vi "Update_Analized_Overlay.vi"(4 "Color":u32(colorbox)=16711680, 6 "Index":i32, 7 "ROI Entry":T11={"vROIName"="", "vROIContour"={"Contour Type"=0, "ROI Type"=0, "Points"=[]}, "ProcessSetting"=[], "Analysis_Setting"={"PreProcess"=enum."*Algorithm*", "Parameter"=""}}, 8 "error in (no error)":errorcluster, 9 "DLL/Vision":bool, 10 "AnalysisResult":variant, 11 "Image Refnum":refnum<vi>) -> (0 "error out":errorcluster, 3 "DLL Vision_Image":T7)   [LabVIEW 2019]
uses:
  DLL/[Global] Image.vi
  <vilib>/vision/NI_Vision_Development_Module.lvlib
  Analysis/Controls/Parttern Match/Analysis_PatternMatch_ResultWithnumber.ctl
  Analysis/Controls/Contour/Analysis_Contour_Result.ctl
  Analysis/Controls/ColorMatch/Analysis_ColorMatch_Result.ctl
  Process/Controls/Process_Setting.ctl
  Analysis/Controls/Analysis_Setting.ctl
  Controls/Vision_DataEntry.ctl
  <vilib>/vision/Measure.llb/Edge New.ctl
  <vilib>/vision/Image Controls.llb/IMAQ Image.ctl
  Ctrl/VisionProcessName.ctl
panel:
  in  "data":T1
  in  "Particle Cluster":T2
  in  "output cluster":T3
  in  "Clamp Cluster":T4={"Points"=[], "Perpendicular Lines"=[], "appended array"=[], "Line Coordinates"=[], "Clamp Settings"={"Contrast"=0, "Filter width"=0, "Steepness"=0, "Subsampling Ratio"=0, "Show Search Area"=FALSE, "Show Search Lines"=FALSE, "Show Edges Found"=FALSE, "Show Result"=FALSE}, "ROI Descriptor"={"Global Rectangle"=[], "Contours"=[]}, "Distance"=0.0, "Edge Coordinates"=[{"X"=441.67966, "Y"=663.0}, {"X"=684.4586, "Y"=655.0}], "Edge Coordinates  (Real World)"=[{"X"=441.67966, "Y"=663.0}, {"X"=684.4586, "Y"=655.0}], "Distance (Real World)"=0.0}
  in  "Edge Detectionoutput cluster":T6 {"Edge Information"."Distance (Real-World)" format="%.2f"; "Edge Information"."Location (Real-World)"."Y" format="%.2g"; "Edge Information"."Location (Real-World)"."X" format="%.2f"; "Edge Information"."Noise" format="%.2f"; "Edge Information"."Location (Pixel)"."Y" format="%.2g"; "Edge Information"."Location (Pixel)"."X" format="%.2f"; "Edge Information"."Strength" format="%.2f"; "Edge Information"."Distance (Pixel)" format="%.2f"}
  in  "Straight Edge Cluster Array":T8(array[cluster])
  in  "Barcode 1D output cluster":T9
  in  "Barcode 2D output cluster":T10
  in  "Vision_Image":T7(plugin-control)
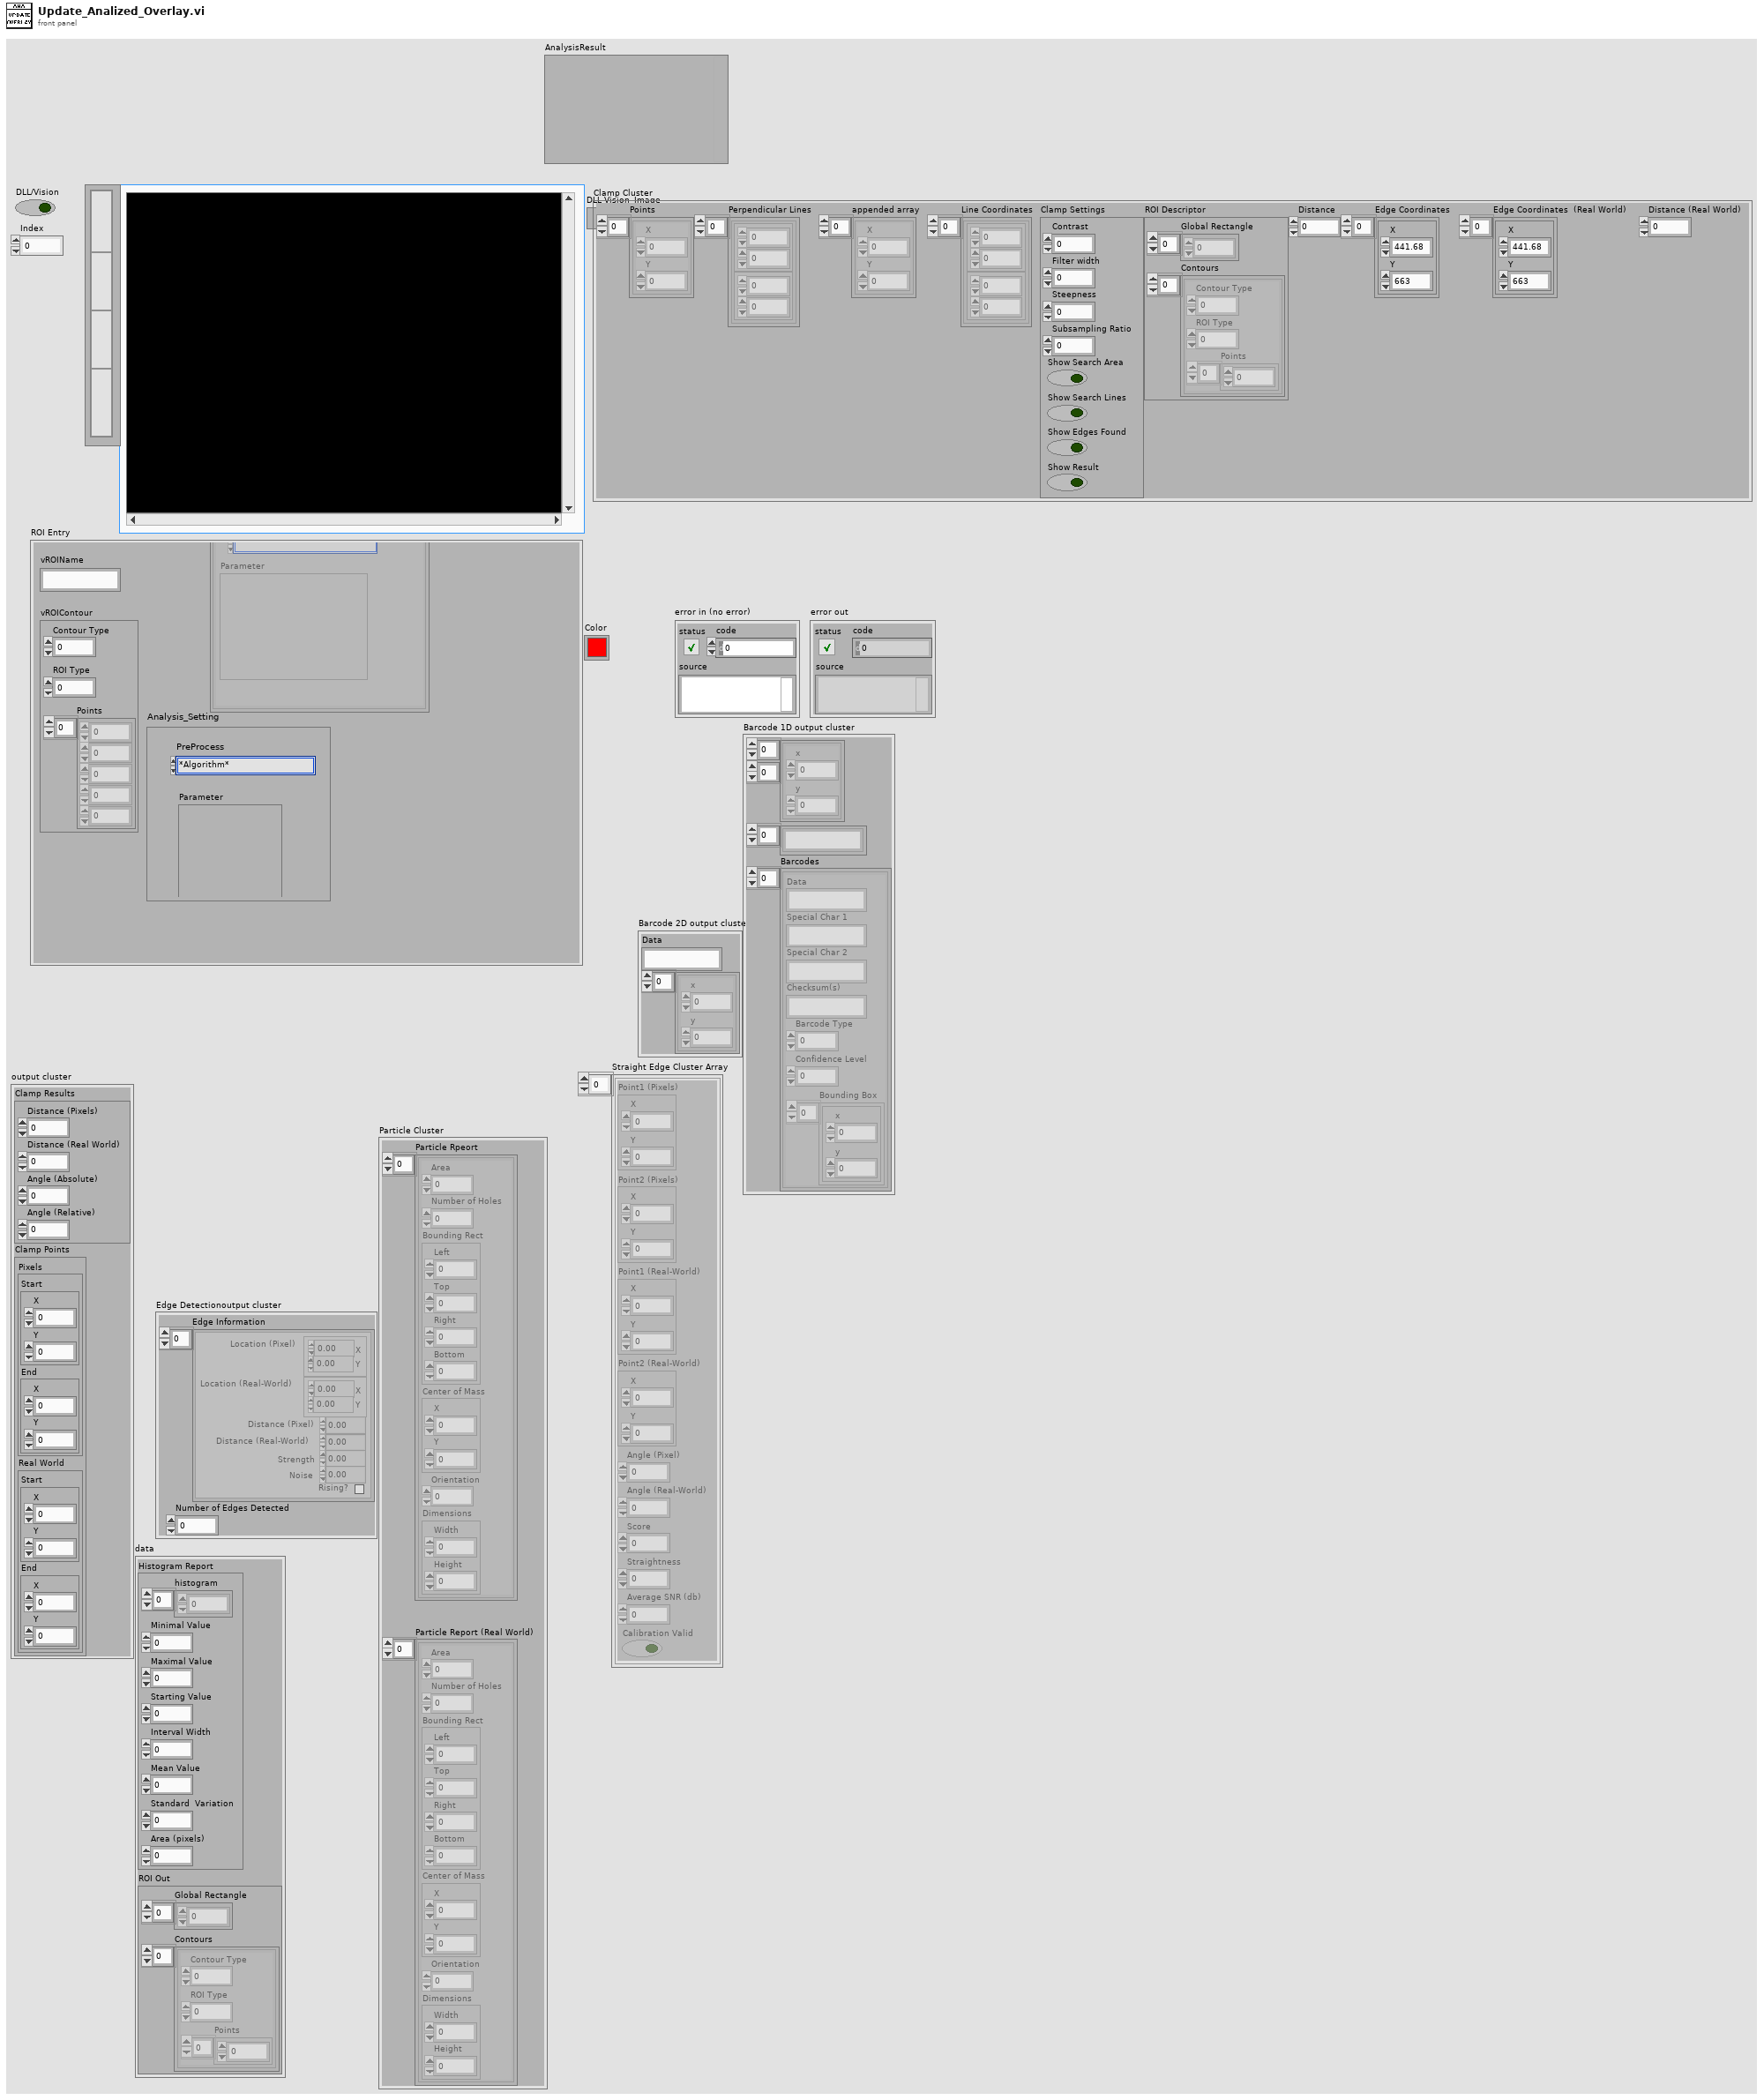
[diagram p1: front panel]
types:
  T1 = cluster{"Histogram Report":cluster{"histogram":u32[], "Minimal Value":sgl, "Maximal Value":sgl, "Starting Value":sgl, "Interval Width":sgl, "Mean Value":sgl, "Standard  Variation":sgl, "Area (pixels)":i32}, "ROI Out":cluster{"Global Rectangle":i32[], "Contours":cluster{"Contour Type":u32, "ROI Type":u32, "Points":i32[]}[]}}
  T2 = cluster{"Particle Rpeort":cluster{"Area":dbl, "Number of Holes":dbl, "Bounding Rect":cluster{"Left":dbl, "Top":dbl, "Right":dbl, "Bottom":dbl}, "Center of Mass":cluster{"X":dbl, "Y":dbl}, "Orientation":dbl, "Dimensions":cluster{"Width":dbl, "Height":dbl}}[], "Particle Report (Real World)":cluster{"Area":dbl, "Number of Holes":dbl, "Bounding Rect":cluster{"Left":dbl, "Top":dbl, "Right":dbl, "Bottom":dbl}, "Center of Mass":cluster{"X":dbl, "Y":dbl}, "Orientation":dbl, "Dimensions":cluster{"Width":dbl, "Height":dbl}}[]}
  T3 = cluster{"Clamp Results":cluster{"Distance (Pixels)":dbl, "Distance (Real World)":dbl, "Angle (Absolute)":dbl, "Angle (Relative)":dbl}, "Clamp Points":cluster{"Pixels ":cluster{"Start":cluster{"X":dbl, "Y":dbl}, "End":cluster{"X":dbl, "Y":dbl}}, "Real World":cluster{"Start":cluster{"X":dbl, "Y":dbl}, "End":cluster{"X":dbl, "Y":dbl}}}}
  T4 = cluster{"Points":cluster{"X":sgl, "Y":sgl}[], "Perpendicular Lines":cluster{cluster{sgl, sgl}, cluster{sgl, sgl}}[], "appended array":cluster{"X":sgl, "Y":sgl}[], "Line Coordinates":cluster{cluster{sgl, sgl}, cluster{sgl, sgl}}[], "Clamp Settings":cluster{"Contrast":i32, "Filter width":i32, "Steepness":i32, "Subsampling Ratio":u32, "Show Search Area":bool, "Show Search Lines":bool, "Show Edges Found":bool, "Show Result":bool}, "ROI Descriptor":cluster{"Global Rectangle":i32[], "Contours":cluster{"Contour Type":u32, "ROI Type":u32, "Points":i32[]}[]}, "Distance":sgl, "Edge Coordinates":cluster{"X":sgl, "Y":sgl}[], "Edge Coordinates  (Real World)":cluster{"X":sgl, "Y":sgl}[], "Distance (Real World)":sgl}
  T5 = typedef "Edge New.ctl" = cluster{"Location (Pixel)":cluster{"X":sgl, "Y":sgl}, "Location (Real-World)":cluster{"X":sgl, "Y":sgl}, "Distance (Pixel)":dbl, "Distance (Real-World)":dbl, "Strength":dbl, "Noise":dbl, "Rising?":bool}
  T6 = cluster{"Edge Information":T5[], "Number of Edges Detected":i32}
  T7 = typedef "IMAQ Image.ctl" = refnum<image>
  T8 = cluster{"Point1 (Pixels)":cluster{"X":sgl, "Y":sgl}, "Point2 (Pixels)":cluster{"X":sgl, "Y":sgl}, "Point1 (Real-World)":cluster{"X":sgl, "Y":sgl}, "Point2 (Real-World)":cluster{"X":sgl, "Y":sgl}, "Angle (Pixel)":dbl, "Angle (Real-World)":dbl, "Score":dbl, "Straightness":dbl, "Average SNR (db)":dbl, "Calibration Valid":bool}[]
  T9 = cluster{cluster{"x":sgl, "y":sgl}[][], string[], "Barcodes":cluster{"Data":string, "Special Char 1":string, "Special Char 2":string, "Checksum(s)":string, "Barcode Type":u32, "Confidence Level":sgl, "Bounding Box":cluster{"x":sgl, "y":sgl}[]}[]}
  T10 = cluster{"Data":string, cluster{"x":sgl, "y":sgl}[]}
  T11 = typedef "Vision_DataEntry.ctl" = cluster{"vROIName":string, "vROIContour":cluster{"Contour Type":u32, "ROI Type":u32, "Points":i32[]}, "ProcessSetting":T12[], "Analysis_Setting":T14}
  T12 = typedef "Process_Setting.ctl" = cluster{"Enum_PreProcess":T13, "Parameter":string}
  T13 = typedef "VisionProcessName.ctl" = enum16{"*CamParameter*", "CamAttributes", "*Preprocess*", "CG_Brightness", "C_Plane Extraction", "C_Threshold", "G_Lookup Table", "G_Threshold"}
  T14 = typedef "Analysis_Setting.ctl" = cluster{"PreProcess":T15, "Parameter":string}
  T15 = typedef "VisionProcessName.ctl" = enum16{"*CamParameter*", "CamAttributes", "*Preprocess*", "CG_Brightness", "C_Plane Extraction", "C_Threshold", "G_Lookup Table", "G_Threshold", "B_Image Inversion", "*Algorithm*", "CG_Histogram", "C_Color Matching", "C_Color Pattern Matching", "G_PatternMatch", "CG_Find Straight Edge", "CG_Adv. Find Straight Edge", "CG_Find Circular Edge", "G_Max Clamp", "G_Clamp (Rake)", "G_Pattern Matching"}
  T16 = typedef "Analysis_Type.ctl" = u16
  T17 = typedef "Analysis_PatternMatch_ResultWithnumber.ctl" = cluster{"numbers":i32, "results":cluster{"ROI Descriptor out":T18, "Point":T19, "Angle":sgl, "Score":sgl, "Real World Coordinates":cluster{"X":sgl, "Y":sgl}, "Rectangle":T20}[]}
  T18 = typedef "ROI Descriptor" = cluster{"Global Rectangle":i32[], "Contours":cluster{"ID":enum32{"External", "Internal"}, "Type":u32, "Coordinates":i32[]}[]}
  T19 = typedef "IMAQ Point" = cluster{"X":sgl, "Y":sgl}
  T20 = typedef "IMAQ Rectangle" = cluster{"Left":i32, "Top":i32, "Right":i32, "Bottom":i32, "Rotation":dbl}
  T21 = cluster{"ROI Descriptor out":T18, "ROI Descriptor out":T18, "Fitted Circle":cluster{"Center (Pixels)":cluster{"X":sgl, "Y":sgl}, "Radius (Pixels)":dbl, "Center (Real-World)":cluster{"X":sgl, "Y":sgl}, "Radius (Real-World)":dbl, "Roundness (Real-World)":dbl, "Average Strength":dbl, "Average SNR (dB)":dbl}}
  T22 = cluster{"Desired Font (Application)":enum16{"User-specified Font", "Application Font", "System Font", "Dialog Font"}, "[User-specified Font]":cluster{"Font Name":string, "Size":i16, "Strikeout?":bool, "Italic?":bool, "Underline?":bool, "Outline?":bool, "Shadow?":bool, "Bold?":bool, "Rotation Angle":dbl}, "Horizontal Alignment":i16, "Vertical Alignment":i16}
  T23 = typedef "Analysis_Contour_Result.ctl" = cluster{"Points (pixel)":cluster{"X":dbl, "Y":dbl}[], "Points (real)":cluster{"X":dbl, "Y":dbl}[], "Length (pixel)":dbl, "Length (real)":dbl}
  T24 = typedef "Analysis_ColorMatch_Result.ctl" = cluster{"Match Flag":bool[], "Match Score":i32[], "ROI Descriptor":T18}
  T25 = cluster{"ROI Descriptor out":T18, "Point":T19, "Angle":sgl, "Score":sgl, "Real World Coordinates":cluster{"X":sgl, "Y":sgl}, "Rectangle":T20}[]
  T26 = cluster{"Contrast":i32, "Filter width":i32, "Steepness":i32, "Subsampling Ratio":u32, "Show Search Area":bool, "Show Search Lines":bool, "Show Edges Found":bool, "Show Result":bool}
  T27 = cluster{"Global Rectangle":i32[], "Contours":cluster{"Contour Type":u32, "ROI Type":u32, "Points":i32[]}[]}
  T28 = cluster{"Start":cluster{"X":dbl, "Y":dbl}, "End":cluster{"X":dbl, "Y":dbl}}
  T29 = cluster{"End":cluster{"X":dbl, "Y":dbl}, "Start":cluster{"X":dbl, "Y":dbl}}
  T30 = cluster{"Point 1":cluster{"X":sgl, "Y":sgl}, "Point 2":cluster{"X":sgl, "Y":sgl}}
  T31 = cluster{cluster{sgl, sgl}, "End":cluster{"X":dbl, "Y":dbl}}
  T32 = cluster{cluster{sgl, sgl}, "Start":cluster{"X":dbl, "Y":dbl}}
  T33 = cluster{"Point 1":cluster{"X":sgl, "Y":sgl}, "Point 2":cluster{"X":sgl, "Y":sgl}}[]
  T34 = cluster{cluster{"X":dbl, "Y":dbl}, cluster{"X":dbl, "Y":dbl}}
  T35 = cluster{cluster{"X":dbl, "Y":dbl}, "End":cluster{"X":dbl, "Y":dbl}}
  T36 = cluster{cluster{"X":dbl, "Y":dbl}, "Start":cluster{"X":dbl, "Y":dbl}}
  T37 = cluster{cluster{"X":dbl, "Y":dbl}, cluster{"X":dbl, "Y":dbl}}[]
  T38 = cluster{"Area":dbl, "Number of Holes":dbl, "Bounding Rect":cluster{"Left":dbl, "Top":dbl, "Right":dbl, "Bottom":dbl}, "Center of Mass":cluster{"X":dbl, "Y":dbl}, "Orientation":dbl, "Dimensions":cluster{"Width":dbl, "Height":dbl}}[]
  T39 = cluster{"Left":dbl, "Top":dbl, "Right":dbl, "Bottom":dbl}
  T40 = cluster{"Contour Type":u32, "ROI Type":u32, "Points":i32[]}[]
  T41 = cluster{"Contour Type":u32, "ROI Type":u32, "Points":i32[]}
  T42 = cluster{"Enum_ShapeType":enum16{"Circles", "Ellipses", "Lines", "Rectangles"}, "numbers":i32, "ReAnfle":cluster{"Rectangle Descriptor":cluster{"Corners":cluster{"X":sgl, "Y":sgl}[], "Angle":dbl, "Width":dbl, "Height":dbl, "Score":dbl}, "Rectangle Descriptor(Real)":cluster{"Corners":cluster{"X":sgl, "Y":sgl}[], "Angle":dbl, "Width":dbl, "Height":dbl, "Score":dbl}}[]}
  T43 = cluster{"Enum_ShapeType":enum16{"Circles", "Ellipses", "Lines", "Rectangles"}, "numbers":i32, "Lines":cluster{"Circle Descriptor":cluster{"Start Point":cluster{"X":sgl, "Y":sgl}, "End Point":cluster{"X":sgl, "Y":sgl}, "Length":dbl, "Angle":dbl, "Score":dbl}, "Circle Descriptor(Real)":cluster{"Start Point":cluster{"X":sgl, "Y":sgl}, "End Point":cluster{"X":sgl, "Y":sgl}, "Length":dbl, "Orientation":dbl, "Score":dbl}}[]}
  T44 = cluster{"Enum_ShapeType":enum16{"Circles", "Ellipses", "Lines", "Rectangles"}, "numbers":i32, "Ellipse":cluster{"ROI Descriptor out":T18, "Circle Descriptor":cluster{"Position":cluster{"X":sgl, "Y":sgl}, "Angle":dbl, "Major Radius":dbl, "Minor Radius":dbl, "Score":dbl}, "Circle Descriptor(Real)":cluster{"Position":cluster{"X":sgl, "Y":sgl}, "Orientation":dbl, "Major Radius":dbl, "Minor Radius":dbl, "Score":dbl}}[]}
  T45 = cluster{"Enum_ShapeType":enum16{"Circles", "Ellipses", "Lines", "Rectangles"}, "numbers":i32, "Circle ":cluster{"ROI Descriptor out":T18, "Circle Descriptor":cluster{"Position":cluster{"X":sgl, "Y":sgl}, "Radius":dbl, "Score":dbl}, "Circle Descriptor(Real)":cluster{"Position":cluster{"X":sgl, "Y":sgl}, "Radius":dbl, "Score":dbl}}[]}
  T46 = cluster{"ROI Descriptor out":T18, "Circle Descriptor":cluster{"Position":cluster{"X":sgl, "Y":sgl}, "Radius":dbl, "Score":dbl}, "Circle Descriptor(Real)":cluster{"Position":cluster{"X":sgl, "Y":sgl}, "Radius":dbl, "Score":dbl}}[]
  T47 = cluster{"ROI Descriptor out":T18, "Circle Descriptor":cluster{"Position":cluster{"X":sgl, "Y":sgl}, "Angle":dbl, "Major Radius":dbl, "Minor Radius":dbl, "Score":dbl}, "Circle Descriptor(Real)":cluster{"Position":cluster{"X":sgl, "Y":sgl}, "Orientation":dbl, "Major Radius":dbl, "Minor Radius":dbl, "Score":dbl}}[]
  T48 = cluster{"Position":cluster{"X":sgl, "Y":sgl}, "Angle":dbl, "Major Radius":dbl, "Minor Radius":dbl, "Score":dbl}
  T49 = cluster{dbl, dbl, "Major Radius":dbl, "Minor Radius":dbl}
  T50 = cluster{"Circle Descriptor":cluster{"Start Point":cluster{"X":sgl, "Y":sgl}, "End Point":cluster{"X":sgl, "Y":sgl}, "Length":dbl, "Angle":dbl, "Score":dbl}, "Circle Descriptor(Real)":cluster{"Start Point":cluster{"X":sgl, "Y":sgl}, "End Point":cluster{"X":sgl, "Y":sgl}, "Length":dbl, "Orientation":dbl, "Score":dbl}}[]
  T51 = cluster{"Start Point":cluster{"X":sgl, "Y":sgl}, "End Point":cluster{"X":sgl, "Y":sgl}, "Length":dbl, "Angle":dbl, "Score":dbl}
  T52 = cluster{"Rectangle Descriptor":cluster{"Corners":cluster{"X":sgl, "Y":sgl}[], "Angle":dbl, "Width":dbl, "Height":dbl, "Score":dbl}, "Rectangle Descriptor(Real)":cluster{"Corners":cluster{"X":sgl, "Y":sgl}[], "Angle":dbl, "Width":dbl, "Height":dbl, "Score":dbl}}[]
  T53 = cluster{"Corners":cluster{"X":sgl, "Y":sgl}[], "Angle":dbl, "Width":dbl, "Height":dbl, "Score":dbl}
  T54 = cluster{"ID":enum32{"External", "Internal"}, "Type":u32, "Coordinates":i32[]}[]
  T55 = cluster{"Coordinates[0]":i32, "Coordinates[1]":i32}
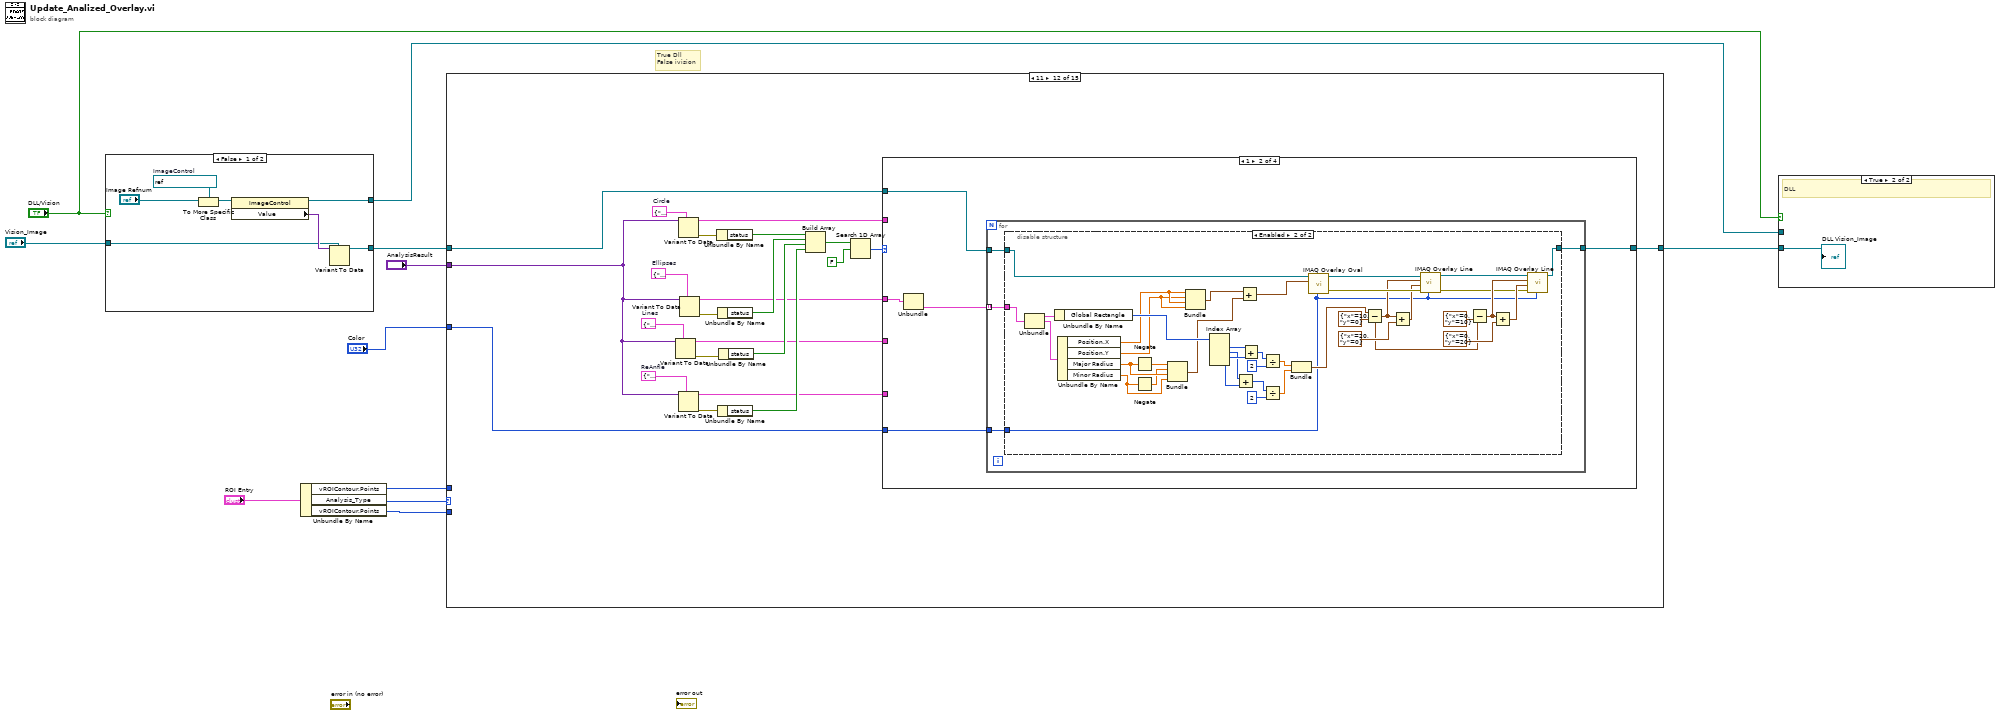
[diagram p0: block diagram]
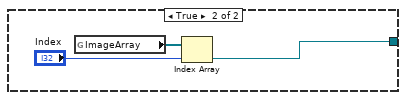
[diagram p2: hidden frame]
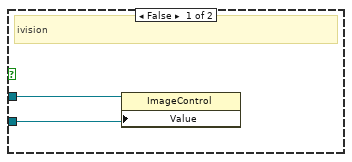
[diagram p3: hidden frame]
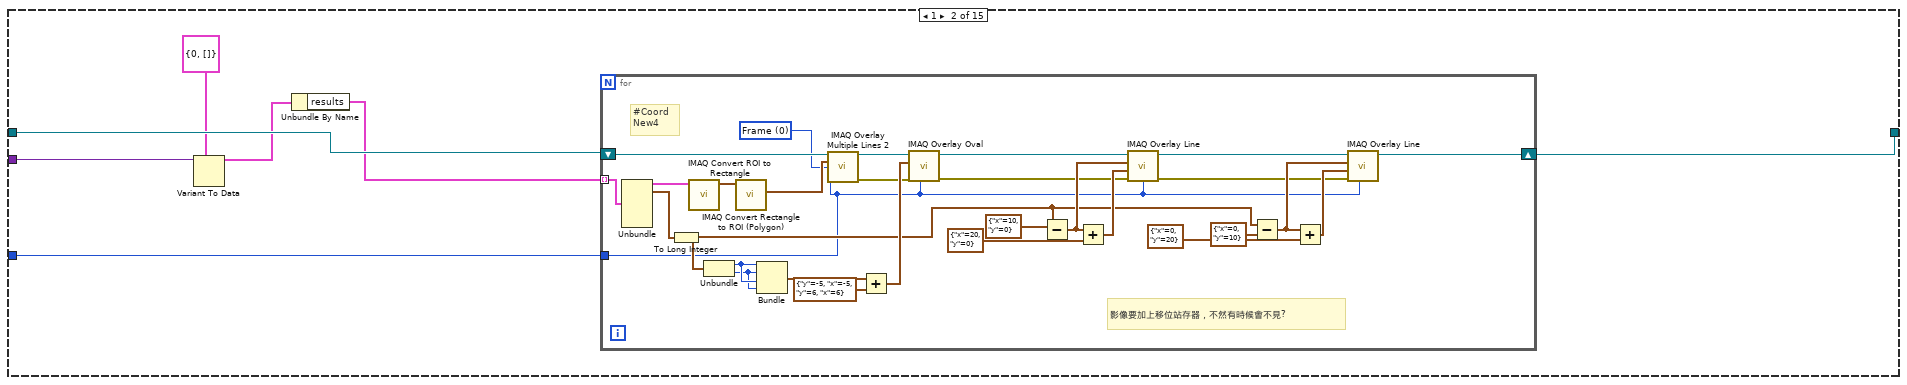
[diagram p5: hidden frame]
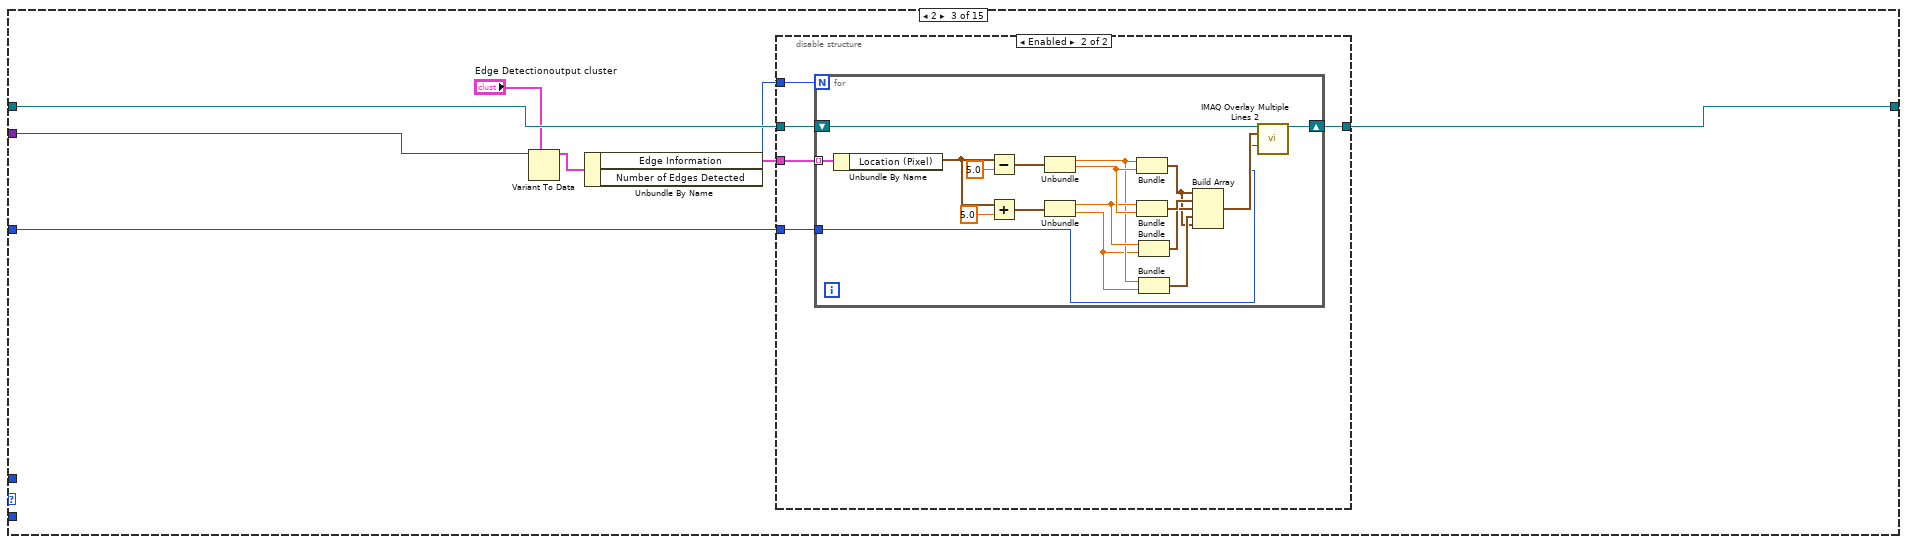
[diagram p6: hidden frame]
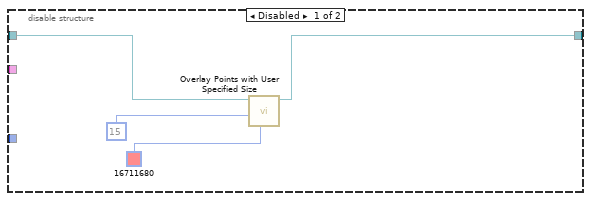
[diagram p7: hidden frame]
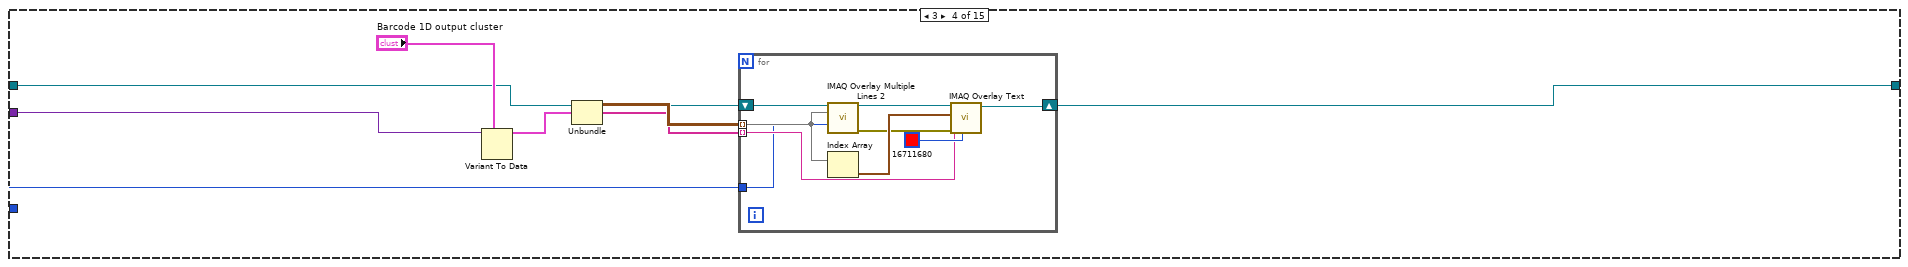
[diagram p8: hidden frame]
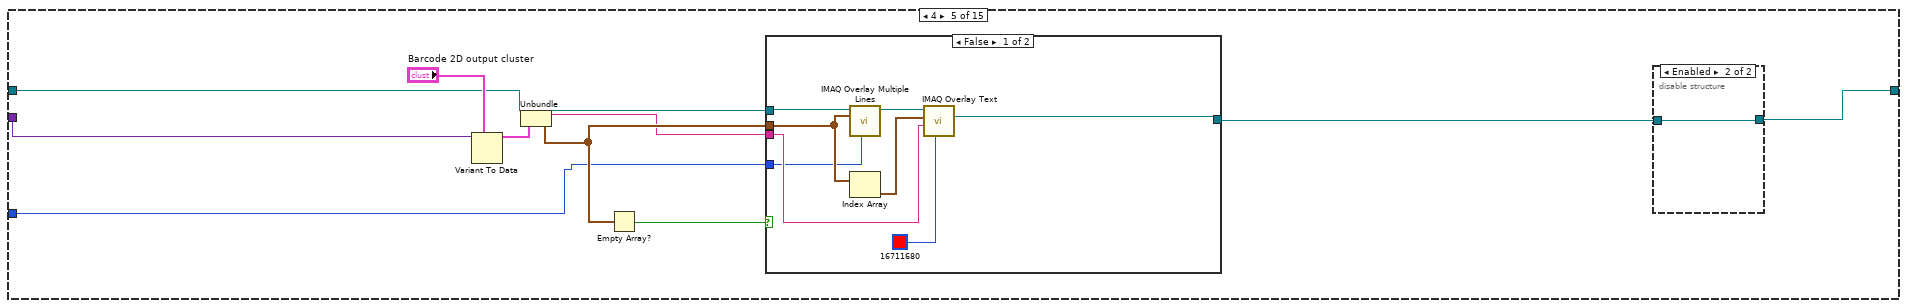
[diagram p9: hidden frame]
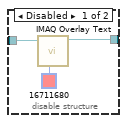
[diagram p11: hidden frame]
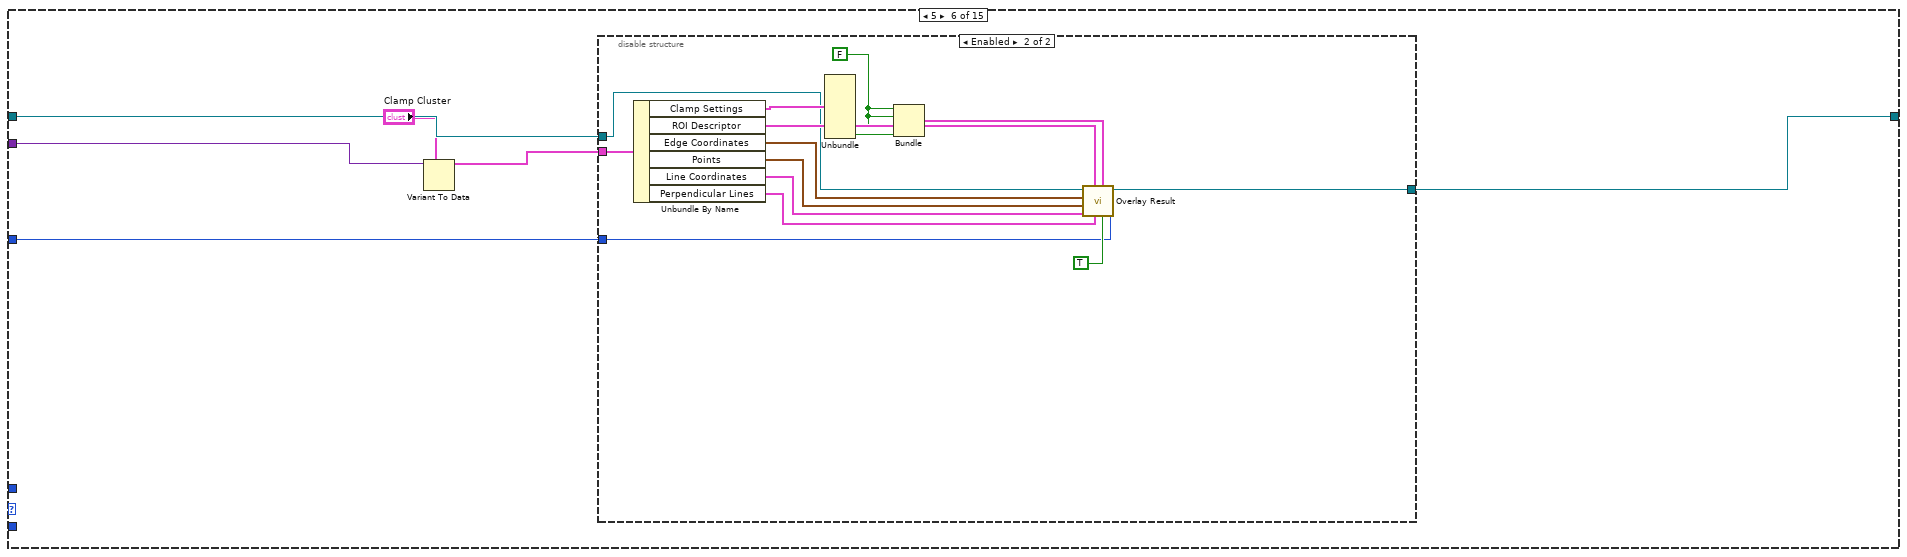
[diagram p12: hidden frame]
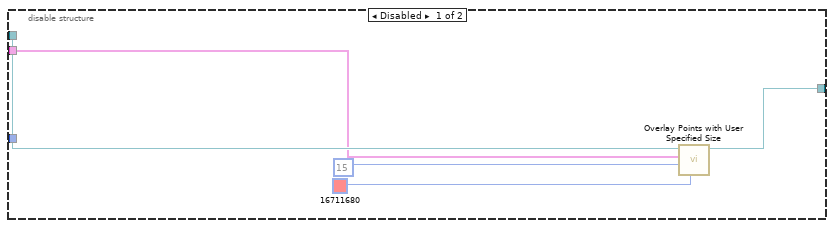
[diagram p13: hidden frame]
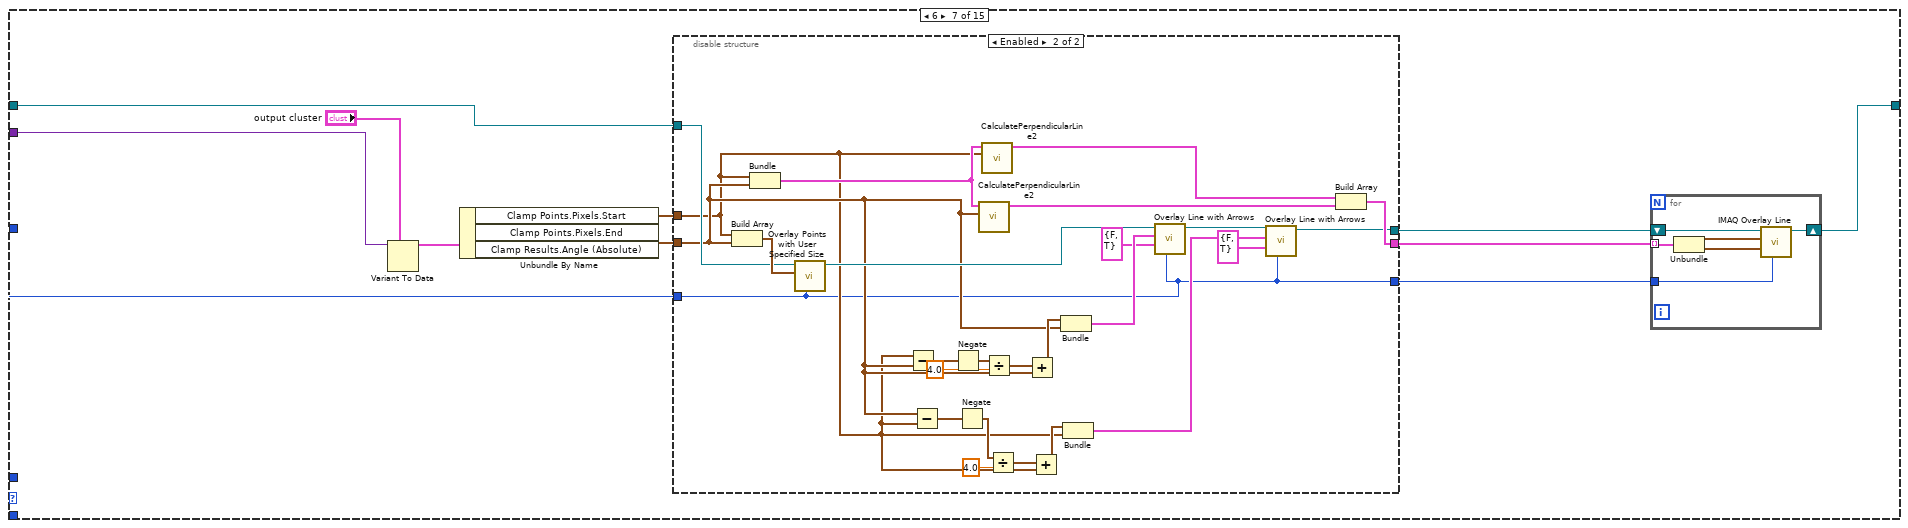
[diagram p14: hidden frame]
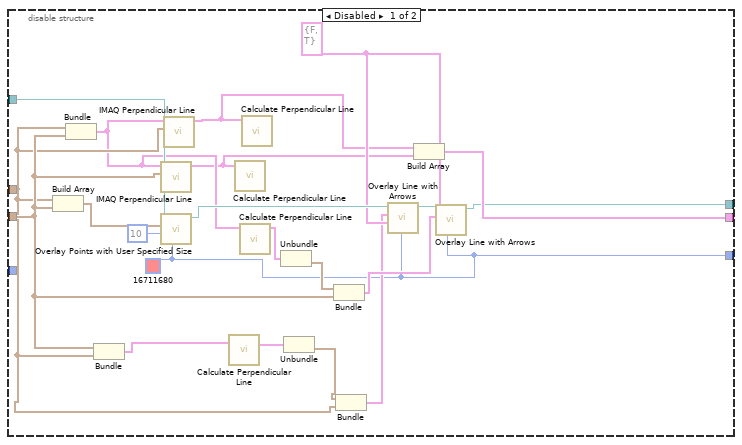
[diagram p15: hidden frame]
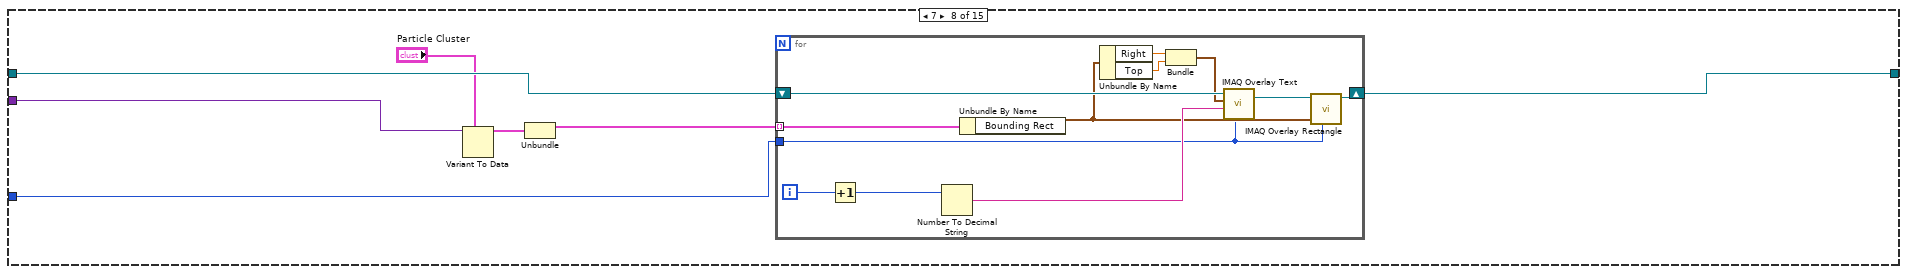
[diagram p16: hidden frame]
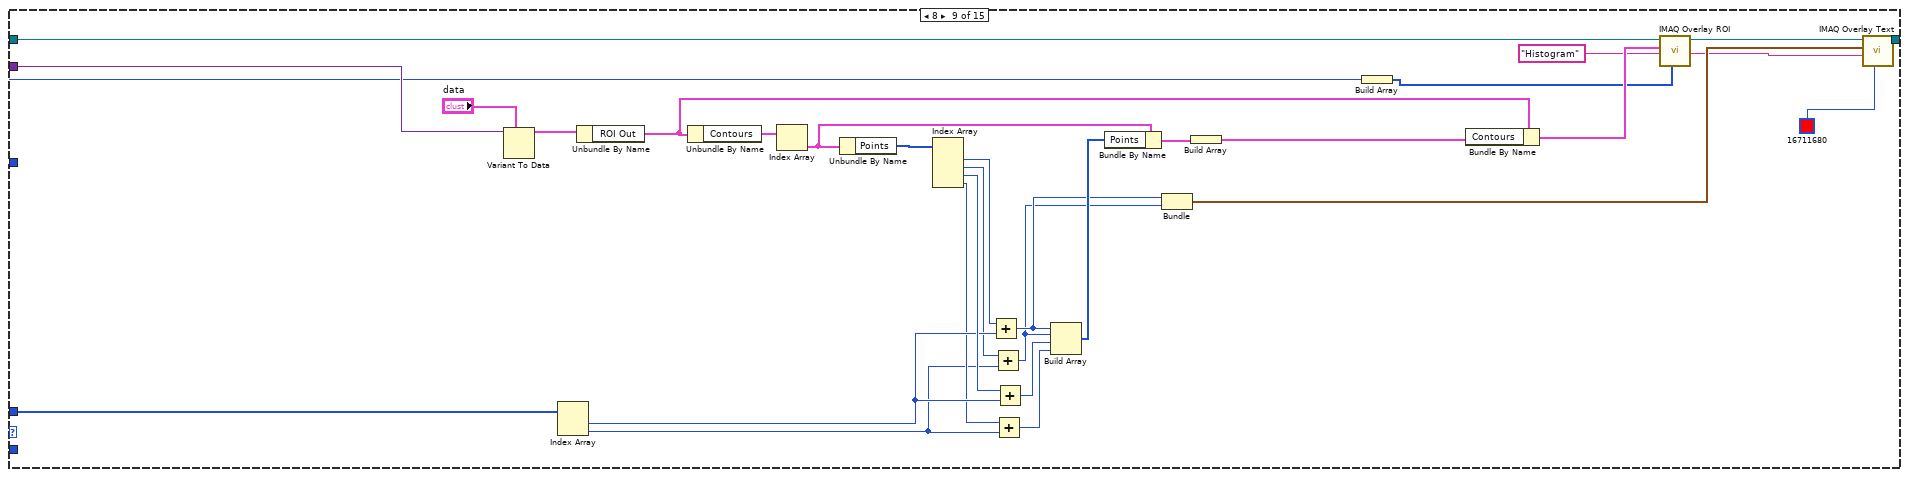
[diagram p17: hidden frame]
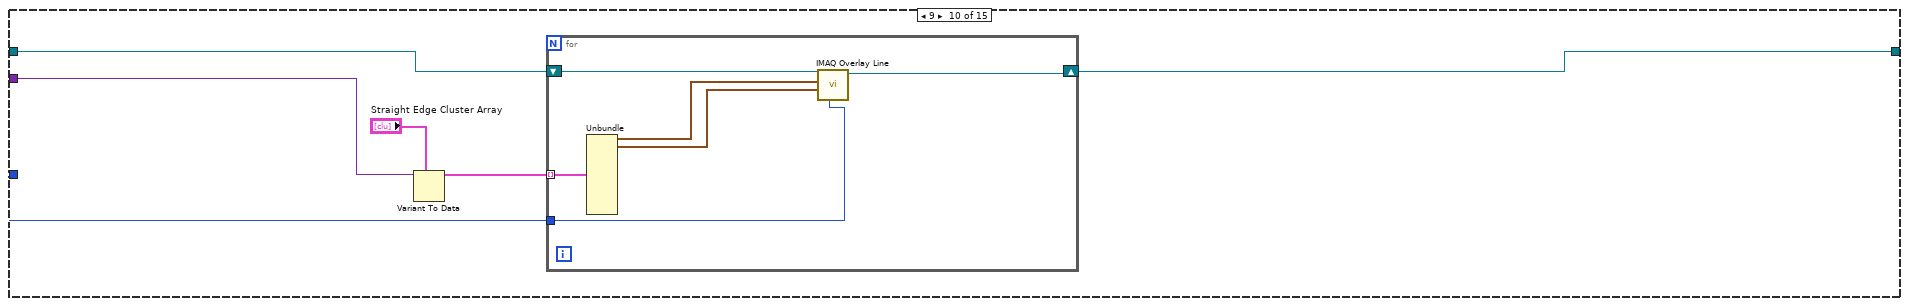
[diagram p18: hidden frame]
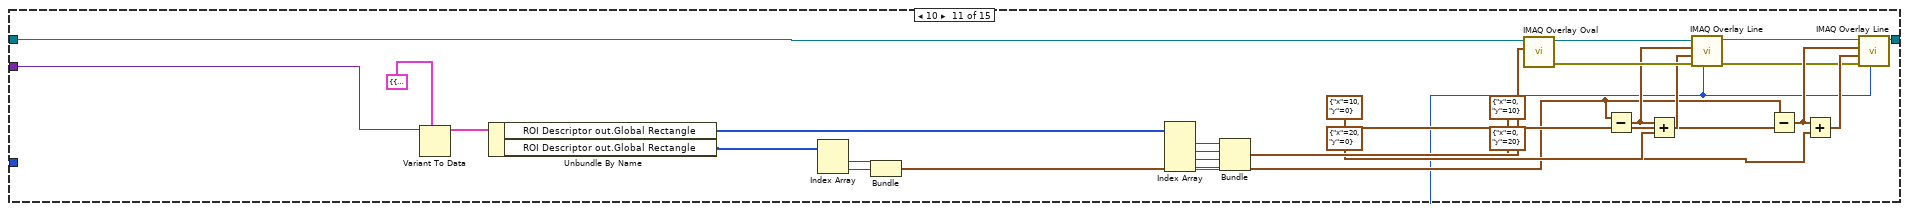
[diagram p19: hidden frame]
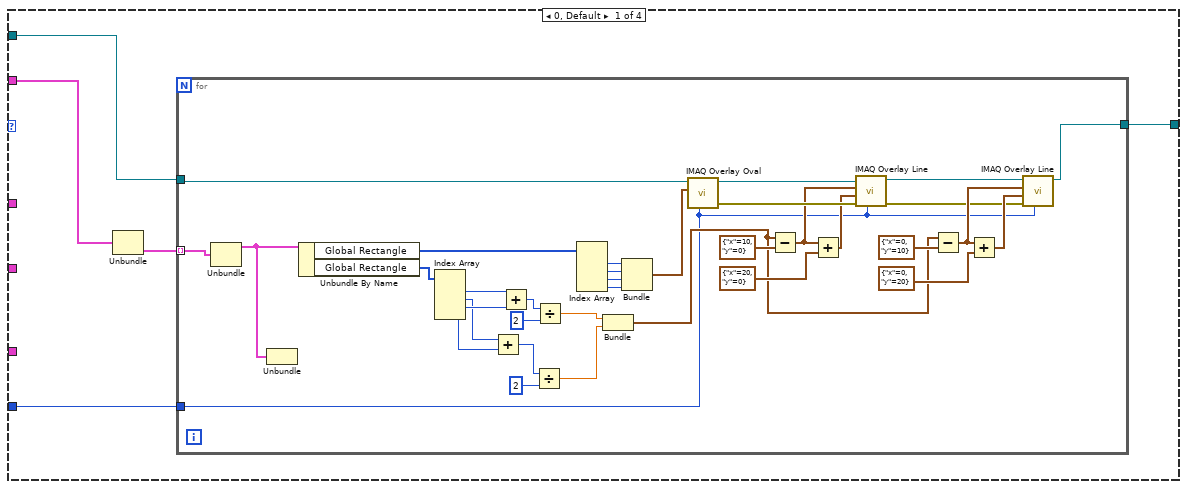
[diagram p20: hidden frame]
diagram:
  # "True Dll\nFalse ivision"
  n1 = case shown="False" "DLL/Vision" {
    tunnel: [w15 _] -> w6
    tunnel: [w13 w19] -> w5
    tunnel: "Vision_Image" -> [w12 _]
    frame False {
      w17 = refnum<vi> refnum  # ImageControl
      n2 = To More Specific Class(target class=w17, reference="Image Refnum") -> (specific class reference=w16:refnum<vi>)  [unwired: 1 in, 1 out]
      n3 = property class="ImageControl"(reference=w16) -> (reference out=w15:refnum<vi>, "Value"=w14:variant)  [unwired: 1 in, 1 out]
      n4 = Variant To Data(type=w12, Variant=w14) -> (data=w13:T7)  [unwired: 1 in, 1 out]
    }
    frame True {
      n5 = global read "[Global] Image.vi" "ImageArray"() -> (w21:T7[])
      n6 = Index Array(array=w21, index="Index") -> (element=w19:T7)
    }
  }
  n7 = Unbundle By Name("ROI Entry") -> ("vROIContour.Points"=w9:i32[], "Analysis_Type"=w8:T16, "vROIContour.Points"=w2:i32[])
  n8 = case shown="11" w8 {
    tunnel: "AnalysisResult" -> [_ w29 w66 w102 w121 w140 w170 w230 w272 w278 w312 w335 w466 w477 w490]
    tunnel: w9 -> [_ _ _ _ _ _ _ _ w271 _ _ _ _ _ _]
    tunnel: [w22 w28 w65 w97 w117 w139 w166 w229 w255 w275 w303 w321 w467 w470 w480] -> w11
    tunnel: w5 -> [w22 w27 w64 w96 w113 w137 w169 w227 w270 w274 w306 w322 w456 w472 w482]
    tunnel: w2 -> [_ _ _ _ _ _ _ _ _ _ _ _ w462 _ _]
    tunnel: "Color" -> [_ w23 w59 w95 w112 w135 w160 w224 w244 w273 w285 w313 w453 w468 w479]
    frame 0, Default {
    }
    frame 1 {
      n9 = Variant To Data(type=T17 {"numbers"=0, "results"=[]} ("PatternMatchResult"), Variant=w29) -> (data=w25:T17)  [unwired: 1 in, 1 out]
      n10 = Unbundle By Name(w25) -> ("results"=w24:T25)
      n11 = for {
        tunnel: w24 -> [w54] mode=indexing
        shift-right: [w32] -> w28
        shift-left: w27 -> [w58]
        tunnel: w23 -> [w30]
        w55 = u32 0 items=["Frame", "Fill"] ("Drawing Mode (Frame)")
        # "#Coord\nNew4"
        # "影像要加上移位站存器，不然有時候會不見?"
        n12 = Unbundle(w54) -> ("ROI Descriptor out"=w53:T18, "Point"=w31:T19)  [unwired: 4 out]
        n13 = To Long Integer(number=w31) -> (32bit integer=w36:cluster{"X":i32, "Y":i32})
        n14 = call "IMAQ Convert ROI to Rectangle"("ROI Descriptor"=w53) -> ("Rectangle"=w56:T20)  [unwired: 8 in, 1 out]
        n15 = Unbundle(w36) -> ("X"=w51:i32, "Y"=w50:i32)
        n16 = call "IMAQ Convert Rectangle to ROI (Polygon)"("Rectangle"=w56) -> ("Rectangle Points"=w57:T19[])  [unwired: 7 in, 2 out]
        n17 = Bundle("X"=w51, "Y"=w50, "X"=w51, "Y"=w50) -> (w49:cluster{"X":i32, "Y":i32, "X":i32, "Y":i32})  [unwired: 1 out]
        n18 = call "IMAQ Overlay Multiple Lines 2"("Image"=w58, "Line End Points"=w57, "Drawing Mode (Frame)"=w55, "Color"=w30) -> ("Image Out"=w52:T7, "error out"=w35:errorcluster)  [unwired: 10 in]
        n19 = Add(x=w49, y=cluster{"y":i32, "x":i32, "y":i32, "x":i32} {"y"=-5, "x"=-5, "y"=6, "x"=6}) -> (x+y=w47:cluster{i32, i32, i32, i32})
        n20 = call "IMAQ Overlay Oval"("Color"=w30, "error in (no error)"=w35, "Bounding Rectangle"=w47, "Image"=w52) -> ("error out"=w34:errorcluster, "Image Out"=w33:T7)  [unwired: 6 in]
        n21 = Subtract(x=w36, y=cluster{"x":i32, "y":i32} {"x"=10, "y"=0}) -> (x-y=w45:cluster{i32, i32})
        n22 = Add(x=w45, y=cluster{"x":i32, "y":i32} {"x"=20, "y"=0}) -> (x+y=w43:cluster{i32, i32})
        n23 = call "IMAQ Overlay Line"("Color"=w30, "error in (no error)"=w34, "End Point"=w43, "Start Point"=w45, "Image"=w33) -> ("error out"=w37:errorcluster, "Image Out"=w38:T7)  [unwired: 1 in, 4 out]
        n24 = Subtract(x=w36, y=cluster{"x":i32, "y":i32} {"x"=0, "y"=10}) -> (x-y=w41:cluster{i32, i32})
        n25 = Add(x=w41, y=cluster{"x":i32, "y":i32} {"x"=0, "y"=20}) -> (x+y=w42:cluster{i32, i32})
        n26 = call "IMAQ Overlay Line"("Color"=w30, "error in (no error)"=w37, "End Point"=w42, "Start Point"=w41, "Image"=w38) -> ("Image Out"=w32:T7)  [unwired: 1 in, 5 out]
      }
    }
    frame 2 {
      n27 = Variant To Data(type="Edge Detectionoutput cluster", Variant=w66) -> (data=w61:T6)  [unwired: 1 in, 1 out]
      n28 = Unbundle By Name(w61) -> ("Edge Information"=w63:T5[], "Number of Edges Detected"=w60:i32)
      n29 = disable-structure shown="Enabled" {
        disable-tunnel: w64 -> [w71 w75]
        disable-tunnel: [w69 w76] -> w65
        disable-tunnel: w63 -> [_ w74]
        disable-tunnel: w60 -> [_ w73]
        disable-tunnel: w59 -> [_ w72]
        frame Disabled {
          n30 = call "Overlay Points with User Specified Size.vi"("Color"=u32 16711680, "Point Diameter (5)"=u32 15, "Image In"=w71) -> ("Image Out"=w69:T7, "Points"=w67:cluster{"X":i32, "Y":i32}[])  [unwired: 6 in, 1 out]
        }
        frame Enabled {
          n31 = for {
            N: w73 -> [_]
            shift-right: [w94] -> w76
            shift-left: w75 -> [w93]
            tunnel: w74 -> [w92] mode=indexing
            tunnel: w72 -> [w77]
            n32 = Unbundle By Name(w92) -> ("Location (Pixel)"=w91:cluster{"X":sgl, "Y":sgl})
            n33 = Subtract(x=w91, y=5.0) -> (x-y=w88:cluster{"X":dbl, "Y":dbl})
            n34 = Add(x=w91, y=5.0) -> (x+y=w87:cluster{"X":dbl, "Y":dbl})
            n35 = Unbundle(w88) -> ("X"=w84:dbl, "Y"=w86:dbl)
            n36 = Unbundle(w87) -> ("X"=w85:dbl, "Y"=w83:dbl)
            n37 = Bundle("X"=w84, "Y"=w86) -> (w79:cluster{"X":dbl, "Y":dbl})  [unwired: 1 in]
            n38 = Bundle("X"=w85, "Y"=w86) -> (w82:cluster{"X":dbl, "Y":dbl})  [unwired: 1 in]
            n39 = Bundle("X"=w85, "Y"=w83) -> (w81:cluster{"X":dbl, "Y":dbl})  [unwired: 1 in]
            n40 = Bundle("X"=w84, "Y"=w83) -> (w80:cluster{"X":dbl, "Y":dbl})  [unwired: 1 in]
            n41 = Build Array(w79, w82, w81, w80, w79) -> (w78:cluster{"X":dbl, "Y":dbl}[])
            n42 = call "IMAQ Overlay Multiple Lines 2"("Image"=w93, "Line End Points"=w78, "Color"=w77) -> ("Image Out"=w94:T7)  [unwired: 11 in, 1 out]
          }
        }
      }
    }
    frame 3 {
      n43 = Variant To Data(type="Barcode 1D output cluster", Variant=w102) -> (data=w100:T9)  [unwired: 1 in, 1 out]
      n44 = Unbundle(w100) -> (w99:cluster{"x":sgl, "y":sgl}[][], w98:string[])  [unwired: 1 out]
      n45 = for {
        tunnel: w99 -> [w106] mode=indexing
        shift-right: [w104] -> w97
        shift-left: w96 -> [w107]
        tunnel: w98 -> [w105] mode=indexing
        tunnel: w95 -> [w103]
        n46 = call "IMAQ Overlay Multiple Lines 2"("Image"=w107, "Line End Points"=w106, "Color"=w103) -> ("Image Out"=w108:T7, "error out"=w110:errorcluster)  [unwired: 11 in]
        n47 = Index Array(array=w106) -> (element=w111:cluster{"x":sgl, "y":sgl})  [unwired: 1 in]
        n48 = call "IMAQ Overlay Text"("Text Color (black)"=u32 16711680, "error in (no error)"=w110, "String"=w105, "Origin"=w111, "Image"=w108) -> ("Image Out"=w104:T7)  [unwired: 5 in, 1 out]
      }
    }
    frame 4 {
      n49 = Variant To Data(type="Barcode 2D output cluster", Variant=w121) -> (data=w119:T10)  [unwired: 1 in, 1 out]
      n50 = Unbundle(w119) -> ("Data"=w114:string, w116:cluster{"x":sgl, "y":sgl}[])
      n51 = Empty Array?(array=w116) -> (empty?=w115:bool)
      n52 = case shown="False" w115 {
        tunnel: [w128 w130] -> w118
        tunnel: w116 -> [w126 _]
        tunnel: w114 -> [w127 _]
        tunnel: w113 -> [w123 w130]
        tunnel: w112 -> [w122 _]
        frame False {
          n53 = call "IMAQ Overlay Multiple Lines"("Color"=w122, "Line End Points"=w126, "Image"=w123) -> ("Image Out"=w129:T7)  [unwired: 7 in, 1 out]
          n54 = Index Array(array=w126) -> (element=w125:cluster{"x":sgl, "y":sgl})  [unwired: 1 in]
          n55 = call "IMAQ Overlay Text"("Text Color (black)"=u32 16711680, "String"=w127, "Origin"=w125, "Image"=w129) -> ("Image Out"=w128:T7)  [unwired: 6 in, 1 out]
        }
        frame True {
        }
      }
      n56 = disable-structure shown="Enabled" {
        disable-tunnel: w118 -> [w132 w134]
        disable-tunnel: [w131 w134] -> w117
        frame Disabled {
          n57 = call "IMAQ Overlay Text"("Text Color (black)"=u32 16711680, "Image"=w132) -> ("Image Out"=w131:T7)  [unwired: 8 in, 1 out]
        }
        frame Enabled {
        }
      }
    }
    frame 5 {
      n58 = Variant To Data(type="Clamp Cluster", Variant=w140) -> (data=w138:T4)  [unwired: 1 in, 1 out]
      n59 = disable-structure shown="Enabled" {
        disable-tunnel: w137 -> [w143 w147]
        disable-tunnel: [w142 w159] -> w139
        disable-tunnel: w138 -> [w141 w148]
        disable-tunnel: w135 -> [_ w146]
        frame Disabled {
          n60 = call "Overlay Points with User Specified Size.vi"("Color"=u32 16711680, "Point Diameter (5)"=u32 15, "Points"=w141, "Image In"=w143) -> ("Image Out"=w142:T7)  [unwired: 6 in, 1 out]
        }
        frame Enabled {
          w150 = FALSE
          n61 = Unbundle By Name(w148) -> ("Clamp Settings"=w153:T26, "ROI Descriptor"=w154:T27, "Edge Coordinates"=w151:cluster{"X":sgl, "Y":sgl}[], "Points"=w155:cluster{"X":sgl, "Y":sgl}[], "Line Coordinates"=w156:cluster{cluster{sgl, sgl}, cluster{sgl, sgl}}[], "Perpendicular Lines"=w157:cluster{cluster{sgl, sgl}, cluster{sgl, sgl}}[])
          n62 = Unbundle(w153) -> ("Show Result"=w149:bool)  [unwired: 7 out]
          n63 = Bundle(w150, w150, w150, "Show Result"=w149) -> (w152:cluster{bool, bool, bool, "Show Result":bool})  [unwired: 1 in]
          n64 = call "Overlay Result.vi"("Search Lines Color"=w146, "Min / Max"=TRUE, "Setup"=w152, "Perpendicular Lines"=w157, "ROI Descriptor"=w154, "Search Lines"=w156, "All Edges Found"=w155, "Measurement Edges"=w151, "Image In"=w147) -> ("Image Out"=w159:T7)  [unwired: 2 in]
        }
      }
    }
    frame 6 {
      n65 = Variant To Data(type="output cluster", Variant=w170) -> (data=w167:T3)  [unwired: 1 in, 1 out]
      n66 = Unbundle By Name(w167) -> ("Clamp Points.Pixels.Start"=w162:cluster{"X":dbl, "Y":dbl}, "Clamp Points.Pixels.End"=w163:cluster{"X":dbl, "Y":dbl})  [unwired: 1 out]
      n67 = disable-structure shown="Enabled" {
        disable-tunnel: w169 -> [w191 w216]
        disable-tunnel: [w188 w215] -> w165
        disable-tunnel: [w185 w203] -> w164
        disable-tunnel: w163 -> [w179 w196]
        disable-tunnel: w162 -> [w178 w195]
        disable-tunnel: [w174 w192] -> w161
        disable-tunnel: w160 -> [_ w192]
        frame Disabled {
          w181 = cluster{"Start point":bool, "End point":bool} {"Start point"=FALSE, "End point"=TRUE} ("Arrows")
          w174 = u32 16711680 ("Color")
          n68 = Build Array(w178, w179) -> (w190:cluster{"X":dbl, "Y":dbl}[])
          n69 = Bundle("Start"=w178, "End"=w179) -> (w173:T28)  [unwired: 1 in]
          n70 = Bundle("End"=w179, "Start"=w178) -> (w177:T29)  [unwired: 1 in]
          n71 = call "IMAQ Perpendicular Line"("Point"=w179, "Line"=w173) -> ("Perpendicular Line"=w171:T30)  [unwired: 7 in, 2 out]
          n72 = call "Overlay Points with User Specified Size.vi"("Color"=w174, "Point Diameter (5)"=u32 10, "Points"=w190, "Image In"=w191) -> ("Image Out"=w183:T7)  [unwired: 6 in, 1 out]
          n73 = call "IMAQ Perpendicular Line"("Point"=w178, "Line"=w173) -> ("Perpendicular Line"=w172:T30)  [unwired: 7 in, 2 out]
          n74 = call "Calculate Perpendicular Line.vi"("Perpendicular Line"=w177) -> ("Cluster"=w176:cluster{cluster{sgl, sgl}, cluster{sgl, sgl}})  [unwired: 10 in]
          n75 = call "Calculate Perpendicular Line.vi"("Perpendicular Line"=w171) -> ()  [unwired: 10 in, 1 out]
          n76 = call "Calculate Perpendicular Line.vi"("Perpendicular Line"=w173) -> ("Cluster"=w187:cluster{cluster{sgl, sgl}, cluster{sgl, sgl}})  [unwired: 10 in]
          n77 = call "Calculate Perpendicular Line.vi"("Perpendicular Line"=w172) -> ()  [unwired: 10 in, 1 out]
          n78 = Unbundle(w187) -> (w184:cluster{sgl, sgl})  [unwired: 1 out]
          n79 = Unbundle(w176) -> (w175:cluster{sgl, sgl})  [unwired: 1 out]
          n80 = Bundle(w184, "End"=w179) -> (w186:T31)  [unwired: 1 in]
          n81 = Bundle(w175, "Start"=w178) -> (w180:T32)  [unwired: 1 in]
          n82 = call <vilib>:"Overlay Line with Arrows.vi"("Color"=w174, "Arrows"=w181, "Line Coordinates"=w180, "Image In"=w183) -> ("Image Out"=w182:T7)  [unwired: 2 in, 5 out]
          n83 = Build Array(w172, w171) -> (w188:T33)
          n84 = call <vilib>:"Overlay Line with Arrows.vi"("Color"=w174, "Arrows"=w181, "Line Coordinates"=w186, "Image In"=w182) -> ("Image Out"=w185:T7)  [unwired: 2 in, 5 out]
        }
        frame Enabled {
          n85 = Build Array(w195, w196) -> (w217:cluster{"X":dbl, "Y":dbl}[])
          n86 = Bundle("Start"=w195, "End"=w196) -> (w213:T28)  [unwired: 1 in]
          n87 = call "Overlay Points with User Specified Size.vi"("Color"=w192, "Points"=w217, "Image In"=w216) -> ("Image Out"=w211:T7)  [unwired: 7 in, 1 out]
          n88 = Subtract(x=w195, y=w196) -> (x-y=w207:cluster{"X":dbl, "Y":dbl})
          n89 = Subtract(x=w196, y=w195) -> (x-y=w200:cluster{"X":dbl, "Y":dbl})
          n90 = Negate(x=w207) -> (-x=w206:cluster{"X":dbl, "Y":dbl})
          n91 = Negate(x=w200) -> (-x=w201:cluster{"X":dbl, "Y":dbl})
          n92 = call "CalculatePerpendicularLine2.vi"("Start"=w196, "Cluster in"=w213) -> ("Cluster out"=w212:T34)  [unwired: 9 in]
          n93 = call "CalculatePerpendicularLine2.vi"("Start"=w195, "Cluster in"=w213) -> ("Cluster out"=w214:T34)  [unwired: 9 in]
          n94 = Divide(x=w206, y=4.0) -> (x/y=w209:cluster{"X":dbl, "Y":dbl})
          n95 = Divide(x=w201, y=4.0) -> (x/y=w198:cluster{"X":dbl, "Y":dbl})
          n96 = Add(x=w209, y=w196) -> (x+y=w210:cluster{"X":dbl, "Y":dbl})
          n97 = Add(x=w198, y=w195) -> (x+y=w197:cluster{"X":dbl, "Y":dbl})
          n98 = Bundle(w210, "End"=w196) -> (w205:T35)  [unwired: 1 in]
          n99 = Bundle(w197, "Start"=w195) -> (w194:T36)  [unwired: 1 in]
          n100 = call <vilib>:"Overlay Line with Arrows.vi"("Color"=w192, "Arrows"=cluster{"Start point":bool, "End point":bool} {"Start point"=FALSE, "End point"=TRUE}, "Line Coordinates"=w205, "Image In"=w211) -> ("Image Out"=w204:T7)  [unwired: 2 in, 5 out]
          n101 = call <vilib>:"Overlay Line with Arrows.vi"("Color"=w192, "Arrows"=cluster{"Start point":bool, "End point":bool} {"Start point"=FALSE, "End point"=TRUE}, "Line Coordinates"=w194, "Image In"=w204) -> ("Image Out"=w203:T7)  [unwired: 2 in, 5 out]
          n102 = Build Array(w214, w212) -> (w215:T37)
        }
      }
      n103 = for {
        shift-right: [w222] -> w166
        shift-left: w164 -> [w223]
        tunnel: w165 -> [w221] mode=indexing
        tunnel: w161 -> [w218]
        n104 = Unbundle(w221) -> (w220:cluster{"X":dbl, "Y":dbl}, w219:cluster{"X":dbl, "Y":dbl})
        n105 = call "IMAQ Overlay Line"("Color"=w218, "End Point"=w219, "Start Point"=w220, "Image"=w223) -> ("Image Out"=w222:T7)  [unwired: 6 in, 1 out]
      }
    }
    frame 7 {
      n106 = Variant To Data(type="Particle Cluster", Variant=w230) -> (data=w228:T2)  [unwired: 1 in, 1 out]
      n107 = Unbundle(w228) -> ("Particle Rpeort"=w225:T38)  [unwired: 1 out]
      n108 = for {
        shift-right: [w242] -> w229
        shift-left: w227 -> [w237]
        tunnel: w225 -> [w241] mode=indexing
        tunnel: w224 -> [w231]
        i -> [w240]
        n109 = Increment(x=w240) -> (x+1=w238:i32)
        n110 = Number To Decimal String(number=w238) -> (decimal integer string=w239:string)  [unwired: 1 in]
        n111 = Unbundle By Name(w241) -> ("Bounding Rect"=w235:T39)
        n112 = Unbundle By Name(w235) -> ("Right"=w234:dbl, "Top"=w233:dbl)
        n113 = Bundle("Right"=w234, "Top"=w233) -> (w232:cluster{"Right":dbl, "Top":dbl})  [unwired: 1 in]
        n114 = call "IMAQ Overlay Text"("Text Color (black)"=w231, "String"=w239, "Origin"=w232, "Image"=w237) -> ("Image Out"=w236:T7)  [unwired: 6 in, 1 out]
        n115 = call "IMAQ Overlay Rectangle"("Color"=w231, "Rectangle"=w235, "Image"=w236) -> ("Image Out"=w242:T7)  [unwired: 7 in, 1 out]
      }
    }
    frame 8 {
      n116 = Variant To Data(type="data", Variant=w272) -> (data=w260:T1)  [unwired: 1 in, 1 out]
      n117 = Index Array(array=w271) -> (element #1=w267:i32, element #2=w265:i32)  [unwired: 2 in]
      n118 = Unbundle By Name(w260) -> ("ROI Out"=w259:T27)
      n119 = Unbundle By Name(w259) -> ("Contours"=w269:T40)
      n120 = Index Array(array=w269) -> (element=w264:T41)  [unwired: 1 in]
      n121 = Unbundle By Name(w264) -> ("Points"=w247:i32[])
      n122 = Index Array(array=w247) -> (element #1=w254:i32, element #2=w253:i32, element #3=w268:i32, element #4=w266:i32)  [unwired: 4 in]
      n123 = Add(x=w254, y=w267) -> (x+y=w249:i32)
      n124 = Add(x=w253, y=w265) -> (x+y=w248:i32)
      n125 = Add(x=w266, y=w265) -> (x+y=w245:i32)
      n126 = Add(x=w268, y=w267) -> (x+y=w246:i32)
      n127 = Build Array(w249, w248, w246, w245) -> (w263:i32[])
      n128 = Bundle By Name(cluster=w264, "Points"=w263) -> (w262:T41)
      n129 = Bundle(w249, w248) -> (w252:cluster{i32, i32})  [unwired: 1 in]
      n130 = Build Array(w262) -> (w261:T40)
      n131 = Build Array(w244) -> (w243:u32[])
      n132 = Bundle By Name(cluster=w259, "Contours"=w261) -> (w258:T27)
      n133 = call "IMAQ Overlay ROI"("Colors (Green)"=w243, "ROI Descriptor"=w258, "Image"=w270) -> ("Image Out"=w256:T7)  [unwired: 7 in, 1 out]
      n134 = call "IMAQ Overlay Text"("Text Color (black)"=u32 16711680, "String"="Histogram", "Origin"=w252, "Image"=w256) -> ("Image Out"=w255:T7)  [unwired: 6 in, 1 out]
    }
    frame 9 {
      n135 = Variant To Data(type="Straight Edge Cluster Array", Variant=w278) -> (data=w277:T8)  [unwired: 1 in, 1 out]
      n136 = for {
        tunnel: w277 -> [w284] mode=indexing
        shift-right: [w282] -> w275
        shift-left: w274 -> [w283]
        tunnel: w273 -> [w279]
        n137 = Unbundle(w284) -> ("Point1 (Pixels)"=w281:cluster{"X":sgl, "Y":sgl}, "Point2 (Pixels)"=w280:cluster{"X":sgl, "Y":sgl})  [unwired: 8 out]
        n138 = call "IMAQ Overlay Line"("Color"=w279, "End Point"=w280, "Start Point"=w281, "Image"=w283) -> ("Image Out"=w282:T7)  [unwired: 6 in, 1 out]
      }
    }
    frame 10 {
      n139 = Variant To Data(type=T21 {"ROI Descriptor out"={"Global Rectangle"=[], "Contours"=[]}, "ROI Descriptor out"={"Global Rectangle"=[], "Contours"=[]}, "Fitted Circle"={"Center (Pixels)"={"X"=0.0, "Y"=0.0}, "Radius (Pixels)"=0.0, "Center (Real-World)"={"X"=0.0, "Y"=0.0}, "Radius (Real-World)"=0.0, "Roundness (Real-World)"=0.0, "Average Strength"=0.0, "Average SNR (dB)"=0.0}} ("output cluster"), Variant=w312) -> (data=w292:T21)  [unwired: 1 in, 1 out]
      n140 = Unbundle By Name(w292) -> ("ROI Descriptor out.Global Rectangle"=w291:i32[], "ROI Descriptor out.Global Rectangle"=w290:i32[])
      n141 = Index Array(array=w290) -> (element #1=w288:i32, element #2=w289:i32)  [unwired: 2 in]
      n142 = Bundle(w288, w289) -> (w287:cluster{i32, i32})  [unwired: 1 in]
      n143 = Index Array(array=w291) -> (element #1=w311:i32, element #2=w310:i32, element #3=w309:i32, element #4=w308:i32)  [unwired: 4 in]
      n144 = Bundle(w311, w310, w309, w308) -> (w307:cluster{i32, i32, i32, i32})  [unwired: 1 in]
      n145 = call "IMAQ Overlay Oval"("Bounding Rectangle"=w307, "Image"=w306) -> ("error out"=w305:errorcluster, "Image Out"=w304:T7)  [unwired: 8 in]
      n146 = Subtract(x=w287, y=cluster{"x":i32, "y":i32} {"x"=10, "y"=0}) -> (x-y=w301:cluster{i32, i32})
      n147 = Add(x=w301, y=cluster{"x":i32, "y":i32} {"x"=20, "y"=0}) -> (x+y=w299:cluster{i32, i32})
      n148 = call "IMAQ Overlay Line"("Color"=w285, "error in (no error)"=w305, "End Point"=w299, "Start Point"=w301, "Image"=w304) -> ("error out"=w293:errorcluster, "Image Out"=w294:T7)  [unwired: 1 in, 4 out]
      n149 = Subtract(x=w287, y=cluster{"x":i32, "y":i32} {"x"=0, "y"=10}) -> (x-y=w297:cluster{i32, i32})
      n150 = Add(x=w297, y=cluster{"x":i32, "y":i32} {"x"=0, "y"=20}) -> (x+y=w298:cluster{i32, i32})
      n151 = call "IMAQ Overlay Line"("Color"=w285, "error in (no error)"=w293, "End Point"=w298, "Start Point"=w297, "Image"=w294) -> ("Image Out"=w303:T7)  [unwired: 1 in, 5 out]
    }
    frame 11 {
      w314 = T42 {"Enum_ShapeType"=enum."Circles", "numbers"=0, "ReAnfle"=[]}  # ReAnfle
      w315 = T43 {"Enum_ShapeType"=enum."Circles", "numbers"=0, "Lines"=[]}  # Lines
      w316 = T44 {"Enum_ShapeType"=enum."Circles", "numbers"=0, "Ellipse"=[]}  # Ellipses
      w317 = T45 {"Enum_ShapeType"=enum."Circles", "numbers"=0, "Circle "=[]}  # Circle
      n152 = Variant To Data(type=w315, Variant=w335) -> (data=w319:T43, error out=w333:errorcluster)  [unwired: 1 in]
      n153 = Variant To Data(type=w317, Variant=w335) -> (data=w323:T45, error out=w331:errorcluster)  [unwired: 1 in]
      n154 = Variant To Data(type=w314, Variant=w335) -> (data=w318:T42, error out=w334:errorcluster)  [unwired: 1 in]
      n155 = Variant To Data(type=w316, Variant=w335) -> (data=w320:T44, error out=w332:errorcluster)  [unwired: 1 in]
      n156 = Unbundle By Name(w331) -> ("status"=w330:bool)
      n157 = Unbundle By Name(w332) -> ("status"=w329:bool)
      n158 = Unbundle By Name(w334) -> ("status"=w327:bool)
      n159 = Unbundle By Name(w333) -> ("status"=w328:bool)
      n160 = Build Array(w330, w329, w328, w327) -> (w326:bool[])
      n161 = Search 1D Array(1D array=w326, element=FALSE) -> (index of element=w324:i32)  [unwired: 1 in]
      n162 = case shown="1" w324 {
        tunnel: w323 -> [w340 _ _ _]
        tunnel: w322 -> [w339 w378 w433 w445]
        tunnel: [w337 w377 w432 w444] -> w321
        tunnel: w320 -> [_ w380 _ _]
        tunnel: w319 -> [_ _ w431 _]
        tunnel: w318 -> [_ _ _ w443]
        tunnel: w313 -> [w336 w376 w430 w442]
        frame 0, Default {
          n163 = Unbundle(w340) -> ("Circle"=w338:T46)  [unwired: 2 out]
          n164 = for {
            tunnel: w339 -> [w356]
            tunnel: w338 -> [w375] mode=indexing
            tunnel: [w355] -> w337
            tunnel: w336 -> [w342]
            n165 = Unbundle(w375) -> ("ROI Descriptor out"=w341:T18)  [unwired: 2 out]
            n166 = Unbundle(w341) -> ()  [unwired: 2 out]
            n167 = Unbundle By Name(w341) -> ("Global Rectangle"=w357:i32[], "Global Rectangle"=w354:i32[])
            n168 = Index Array(array=w354) -> (element #1=w353:i32, element #2=w351:i32, element #3=w352:i32, element #4=w350:i32)  [unwired: 4 in]
            n169 = Add(x=w351, y=w350) -> (x+y=w346:i32)
            n170 = Add(x=w353, y=w352) -> (x+y=w349:i32)
            n171 = Divide(x=w346, y=2) -> (x/y=w344:dbl)
            n172 = Divide(x=w349, y=2) -> (x/y=w345:dbl)
            n173 = Index Array(array=w357) -> (element #1=w374:i32, element #2=w373:i32, element #3=w372:i32, element #4=w371:i32)  [unwired: 4 in]
            n174 = Bundle(w345, w344) -> (w343:cluster{dbl, dbl})  [unwired: 1 in]
            n175 = Bundle(w374, w373, w372, w371) -> (w370:cluster{i32, i32, i32, i32})  [unwired: 1 in]
            n176 = call "IMAQ Overlay Oval"("Color"=w342, "Bounding Rectangle"=w370, "Image"=w356) -> ("error out"=w369:errorcluster, "Image Out"=w368:T7)  [unwired: 7 in]
            n177 = Subtract(x=w343, y=cluster{"x":i32, "y":i32} {"x"=10, "y"=0}) -> (x-y=w366:cluster{dbl, dbl})
            n178 = Add(x=w366, y=cluster{"x":i32, "y":i32} {"x"=20, "y"=0}) -> (x+y=w364:cluster{dbl, dbl})
            n179 = call "IMAQ Overlay Line"("Color"=w342, "error in (no error)"=w369, "End Point"=w364, "Start Point"=w366, "Image"=w368) -> ("error out"=w358:errorcluster, "Image Out"=w359:T7)  [unwired: 1 in, 4 out]
            n180 = Subtract(x=w343, y=cluster{"x":i32, "y":i32} {"x"=0, "y"=10}) -> (x-y=w362:cluster{dbl, dbl})
            n181 = Add(x=w362, y=cluster{"x":i32, "y":i32} {"x"=0, "y"=20}) -> (x+y=w363:cluster{dbl, dbl})
            n182 = call "IMAQ Overlay Line"("Color"=w342, "error in (no error)"=w358, "End Point"=w363, "Start Point"=w362, "Image"=w359) -> ("Image Out"=w355:T7)  [unwired: 1 in, 5 out]
          }
        }
        frame 1 {
          n183 = Unbundle(w380) -> ("Ellipse"=w379:T47)  [unwired: 2 out]
          n184 = for {
            tunnel: w379 -> [w384] mode=indexing
            tunnel: w378 -> [w383]
            tunnel: [w382] -> w377
            tunnel: w376 -> [w381]
            n185 = disable-structure shown="Enabled" {
              disable-tunnel: w384 -> [w390 w404]
              disable-tunnel: w383 -> [w389 w403]
              disable-tunnel: [w388 w401] -> w382
              disable-tunnel: w381 -> [w386 w402]
              frame Disabled {
                n186 = Unbundle(w390) -> ("ROI Descriptor out"=w387:T18)  [unwired: 2 out]
                n187 = Build Array(w386) -> (w385:u32[])
                n188 = call "IMAQ Overlay ROI"("Colors (Green)"=w385, "ROI Descriptor"=w387, "Image"=w389) -> ("Image Out"=w388:T7)  [unwired: 7 in, 1 out]
              }
              frame Enabled {
                n189 = Unbundle(w404) -> ("ROI Descriptor out"=w417:T18, "Circle Descriptor"=w400:T48)  [unwired: 1 out]
                n190 = Unbundle By Name(w417) -> ("Global Rectangle"=w416:i32[])
                n191 = Unbundle By Name(w400) -> ("Position.X"=w399:sgl, "Position.Y"=w398:sgl, "Major Radius"=w396:dbl, "Minor Radius"=w394:dbl)
                n192 = Negate(x=w396) -> (-x=w397:dbl)
                n193 = Negate(x=w394) -> (-x=w395:dbl)
                n194 = Bundle(w397, w395, "Major Radius"=w396, "Minor Radius"=w394) -> (w392:T49)  [unwired: 1 in]
                n195 = Bundle("X"=w399, "Y"=w398, "X"=w399, "Y"=w398) -> (w393:cluster{"X":sgl, "Y":sgl, "X":sgl, "Y":sgl})  [unwired: 1 in]
                n196 = Index Array(array=w416) -> (element #1=w415:i32, element #2=w413:i32, element #3=w414:i32, element #4=w412:i32)  [unwired: 4 in]
                n197 = Add(x=w413, y=w412) -> (x+y=w408:i32)
                n198 = Add(x=w393, y=w392) -> (x+y=w391:cluster{dbl, dbl, dbl, dbl})
                n199 = Add(x=w415, y=w414) -> (x+y=w411:i32)
                n200 = Divide(x=w411, y=2) -> (x/y=w407:dbl)
                n201 = Divide(x=w408, y=2) -> (x/y=w406:dbl)
                n202 = Bundle(w407, w406) -> (w405:cluster{dbl, dbl})  [unwired: 1 in]
                n203 = call "IMAQ Overlay Oval"("Color"=w402, "Bounding Rectangle"=w391, "Image"=w403) -> ("error out"=w429:errorcluster, "Image Out"=w428:T7)  [unwired: 7 in]
                n204 = Subtract(x=w405, y=cluster{"x":i32, "y":i32} {"x"=10, "y"=0}) -> (x-y=w426:cluster{dbl, dbl})
                n205 = Add(x=w426, y=cluster{"x":i32, "y":i32} {"x"=20, "y"=0}) -> (x+y=w424:cluster{dbl, dbl})
                n206 = call "IMAQ Overlay Line"("Color"=w402, "error in (no error)"=w429, "End Point"=w424, "Start Point"=w426, "Image"=w428) -> ("error out"=w418:errorcluster, "Image Out"=w419:T7)  [unwired: 1 in, 4 out]
                n207 = Subtract(x=w405, y=cluster{"x":i32, "y":i32} {"x"=0, "y"=10}) -> (x-y=w422:cluster{dbl, dbl})
                n208 = Add(x=w422, y=cluster{"x":i32, "y":i32} {"x"=0, "y"=20}) -> (x+y=w423:cluster{dbl, dbl})
                n209 = call "IMAQ Overlay Line"("Color"=w402, "error in (no error)"=w418, "End Point"=w423, "Start Point"=w422, "Image"=w419) -> ("Image Out"=w401:T7)  [unwired: 1 in, 5 out]
              }
            }
          }
        }
        frame 2 {
          n210 = Unbundle(w431) -> ("Lines"=w434:T50)  [unwired: 2 out]
          n211 = for {
            tunnel: w434 -> [w441] mode=indexing
            tunnel: w433 -> [w440]
            tunnel: [w439] -> w432
            tunnel: w430 -> [w435]
            n212 = Unbundle(w441) -> ("Circle Descriptor"=w438:T51)  [unwired: 1 out]
            n213 = Unbundle(w438) -> ("Start Point"=w437:cluster{"X":sgl, "Y":sgl}, "End Point"=w436:cluster{"X":sgl, "Y":sgl})  [unwired: 3 out]
            n214 = call "IMAQ Overlay Line"("Color"=w435, "End Point"=w436, "Start Point"=w437, "Image"=w440) -> ("Image Out"=w439:T7)  [unwired: 6 in, 1 out]
          }
        }
        frame 3 {
          n215 = Unbundle(w443) -> ("ReAnfle"=w446:T52)  [unwired: 2 out]
          n216 = for {
            tunnel: w446 -> [w452] mode=indexing
            tunnel: w445 -> [w451]
            tunnel: [w450] -> w444
            tunnel: w442 -> [w447]
            n217 = Unbundle(w452) -> ("Rectangle Descriptor"=w449:T53)  [unwired: 1 out]
            n218 = Unbundle(w449) -> ("Corners"=w448:cluster{"X":sgl, "Y":sgl}[])  [unwired: 4 out]
            n219 = call "IMAQ Overlay Multiple Lines 2"("Image"=w451, "Line End Points"=w448, "Color"=w447) -> ("Image Out"=w450:T7)  [unwired: 11 in, 1 out]
          }
        }
      }
    }
    frame 12 {
      n220 = Variant To Data(type="", Variant=w466) -> (data=w464:string)  [unwired: 1 in, 1 out]
      n221 = Index Array(array=w462) -> (element #1=w461:i32, element #2=w460:i32, element #3=w459:i32, element #4=w458:i32)  [unwired: 4 in]
      n222 = Bundle(w461, w460) -> (w454:cluster{i32, i32})  [unwired: 1 in]
      n223 = Bundle(w461, w460, w459, w458) -> (w457:cluster{i32, i32, i32, i32})  [unwired: 1 in]
      n224 = call "IMAQ Overlay Rectangle"("Color"=w453, "Rectangle"=w457, "Image"=w456) -> ("Image Out"=w455:T7)  [unwired: 7 in, 1 out]
      n225 = call "IMAQ Overlay Text"("Text Color (black)"=w453, "Font, Size & Style"=T22 {"Desired Font (Application)"=enum."User-specified Font", "[User-specified Font]"={"Font Name"="", "Size"=30, "Strikeout?"=FALSE, "Italic?"=FALSE, "Underline?"=FALSE, "Outline?"=FALSE, "Shadow?"=FALSE, "Bold?"=FALSE, "Rotation Angle"=0.0}, "Horizontal Alignment"=0, "Vertical Alignment"=0}, "String"=w464, "Origin"=w454, "Image"=w455) -> ("Image Out"=w467:T7)  [unwired: 5 in, 1 out]
    }
    frame 13 {
      n226 = Variant To Data(type=T23 {"Points (pixel)"=[], "Points (real)"=[], "Length (pixel)"=0.0, "Length (real)"=0.0} ("ContourResult"), Variant=w477) -> (data=w475:T23, error out=w474:errorcluster)  [unwired: 1 in]
      n227 = call <vilib>:"Clear Errors.vi"("error in (no error)"=w474) -> ("error out"=w473:errorcluster)  [unwired: 5 in, 1 out]
      n228 = Unbundle By Name(w475) -> ("Points (pixel)"=w471:cluster{"X":dbl, "Y":dbl}[])
      n229 = call "IMAQ Overlay Multiple Lines"("Color"=w468, "error in (no error)"=w473, "Line End Points"=w471, "Image"=w472) -> ("error out"=w469:errorcluster, "Image Out"=w470:T7)  [unwired: 6 in]
      n230 = call <vilib>:"Clear Errors.vi"("error in (no error)"=w469) -> ()  [unwired: 5 in, 2 out]
    }
    frame 14 {
      n231 = Variant To Data(type=T24 {"Match Flag"=[], "Match Score"=[], "ROI Descriptor"={"Global Rectangle"=[], "Contours"=[]}} ("output cluster"), Variant=w490) -> (data=w489:T24, error out=w488:errorcluster)  [unwired: 1 in]
      n232 = call <vilib>:"Clear Errors.vi"("error in (no error)"=w488) -> ("error out"=w481:errorcluster)  [unwired: 5 in, 1 out]
      n233 = Unbundle By Name(w489) -> ("Match Flag"=w484:bool[], "ROI Descriptor"=w483:T18)
      n234 = Build Array(w479) -> (w478:u32[])
      n235 = call "IMAQ Overlay ROI"("Colors (Green)"=w478, "ROI Descriptor"=w483, "Image"=w482) -> ("Image Out"=w485:T7)  [unwired: 7 in, 1 out]
      n236 = Unbundle(w483) -> ("Contours"=w486:T54)  [unwired: 1 out]
      n237 = for {
        shift-right: [w494] -> _
        shift-left: w481 -> [w495]
        shift-right: [w493] -> w480
        shift-left: w485 -> [w496]
        tunnel: w484 -> [w492] mode=indexing
        tunnel: w486 -> [w491] mode=indexing
        n238 = case shown="True" w492 {
          tunnel: w496 -> [w501 w510]
          tunnel: w491 -> [w498 w513]
          tunnel: w495 -> [w500 w509]
          tunnel: [w504 w514] -> w493
          tunnel: [w499 w508] -> w494
          frame False {
            # "Use first two coordinates of ROI to make point"
            n239 = Unbundle By Name(w498) -> ("Coordinates"=w497:i32[])
            n240 = Array To Cluster(array=w497) -> (cluster=w503:T55)
            n241 = call "IMAQ Overlay Text"("BG Color (Transparent)"=u32 16711680, "Font, Size & Style"=T22 {"Desired Font (Application)"=enum."Application Font", "[User-specified Font]"={"Font Name"="", "Size"=12, "Strikeout?"=FALSE, "Italic?"=FALSE, "Underline?"=FALSE, "Outline?"=FALSE, "Shadow?"=FALSE, "Bold?"=FALSE, "Rotation Angle"=0.0}, "Horizontal Alignment"=0, "Vertical Alignment"=1}, "error in (no error)"=w500, "String"="FAIL", "Origin"=w503, "Image"=w501) -> ("error out"=w499:errorcluster, "Image Out"=w504:T7)  [unwired: 4 in]
          }
          frame True {
            # "Use first two coordinates of ROI to make point"
            n242 = Unbundle By Name(w513) -> ("Coordinates"=w507:i32[])
            n243 = Array To Cluster(array=w507) -> (cluster=w512:T55)
            n244 = call "IMAQ Overlay Text"("BG Color (Transparent)"=u32 6618880, "Font, Size & Style"=T22 {"Desired Font (Application)"=enum."Application Font", "[User-specified Font]"={"Font Name"="", "Size"=12, "Strikeout?"=FALSE, "Italic?"=FALSE, "Underline?"=FALSE, "Outline?"=FALSE, "Shadow?"=FALSE, "Bold?"=FALSE, "Rotation Angle"=0.0}, "Horizontal Alignment"=0, "Vertical Alignment"=1}, "error in (no error)"=w509, "String"="PASS", "Origin"=w512, "Image"=w510) -> ("error out"=w508:errorcluster, "Image Out"=w514:T7)  [unwired: 4 in]
          }
        }
      }
    }
  }
  n245 = case shown="True" "DLL/Vision" {
    tunnel: w11 -> [w518 w519]
    tunnel: w6 -> [w517 _]
    frame False {
      # "ivision"
      n246 = property class="ImageControl"(reference=w517, "Value"=w518) -> ()  [unwired: 1 in, 2 out]
    }
    frame True {
      # "DLL"
      "DLL Vision_Image" <- w519
    }
  }
